vi "obs2lane.vi"(11 "sensors inputs":dbl[][](array[numeric])=[[-2.6493086559458767, 9.313377271515247, 0.316177936945349, -1.2], [-2.6066100840450477, 9.354542103994737, 0.3157590885476819, -1.2], [-2.579340659822815, 9.43207739327695, 0.31450254335468053, -1.2], [-2.6132527619437576, 9.439068677849818, 0.5859163050429868, 1.2000000000000006], [-2.6655003955140795, 9.41719146151926, 0.4953083793337705, 0.40000000000000013], [-2.8189313467074544, 9.344249551531279, 0.5859163050429868, 1.2000000000000006], [-2.5692189092921667, 9.480018973387281, 0.5863351534406539, 1.2000000000000006], [-2.6731933264342116, 9.434269134901442, 0.5863351534406539, 1.2000000000000006], [-2.77635346299322, 9.386711660550553, 0.5863351534406539, 1.2000000000000006], [-2.7290628288714722, 9.419794899689457, 0.5865445776394874, 1.2000000000000006], [-3.035140869949269, 9.26885391372332, 0.5865445776394874, 1.2000000000000006], [-2.550914688564252, 9.509578404068655, 0.3132459981616791, -1.2], [-2.785425991035746, 9.405948172518677, 0.495587629745689, 0.40000000000000013], [-2.7463409502228373, 9.457274042188466, 0.4957970675546278, 0.40000000000000013], [-2.90576588154835, 9.392310316924437, 0.49586688015760744, 0.40000000000000013], [-2.494747129058042, 9.597974241579312, 0.5880105470313224, 1.2000000000000006], [-2.836998990617639, 9.447892074399023, 0.4039934946364334, -0.3999999999999999], [-3.1184925197733824, 9.303796817000539, 0.5880105470313224, 1.2000000000000006], [-2.970577318209098, 9.393517402151646, 0.4960763179665463, 0.40000000000000013], [-2.9699981982750367, 9.392368449256733, 0.588219971230156, 1.2000000000000006], [-3.0729809459427746, 9.340776068194645, 0.4960763179665463, 0.40000000000000013], [-3.1996655181339673, 9.27234939560896, 0.40392368203345375, -0.3999999999999999], [-3.4973819131319495, 9.096981036828707, 0.40392368203345375, -0.3999999999999999], [-2.5289827185611418, 9.605504378157487, 0.3115706045710105, -1.2], [-3.453631348161608, 9.135814142218397, 0.4038538694304742, -0.3999999999999999], [-3.2339632015510937, 9.274656811335685, 0.5886388196278232, 1.2000000000000006], [-2.483097010676977, 9.64588076688389, 0.3111517561733434, -1.2], [-2.8803018639560647, 9.47148380231442, 0.4962857557754851, 0.40000000000000013], [-2.9317308980723027, 9.444962161904348, 0.5888482438266567, 1.2000000000000006], [-2.9582194094409178, 9.433270224287725, 0.4037142442245149, -0.3999999999999999], [-3.0350382771601945, 9.392890956174119, 0.5888482438266567, 1.2000000000000006], [-2.4599617564514022, 9.665942841266034, 0.5890576680254903, 1.2000000000000006], [-3.1930649800894275, 9.320188914278454, 0.5890576680254903, 1.2000000000000006], [-3.424919733239901, 9.200023640728578, 0.4035746190185557, -0.3999999999999999], [-3.4490855593711203, 9.183917089574846, 0.5892670922243238, 1.2000000000000006], [-2.6822275888719656, 9.595825896338217, 0.49649519358442396, 0.40000000000000013], [-3.1777999006997932, 9.352779338748892, 0.40350480641557607, -0.3999999999999999], [-3.3543988506422, 9.251882705008573, 0.5894765164231575, 1.2000000000000006], [-2.4169315260491846, 9.715129108585124, 0.589685940621991, 1.2000000000000006], [-2.4440270491484113, 9.70452412526726, 0.3103140593780091, -1.2], [-2.4445036099706936, 9.705733945395902, 0.40343499381259645, -0.3999999999999999], [-2.8187951120879293, 9.544925625371082, 0.40343499381259645, -0.3999999999999999], [-2.923864294836344, 9.494810195959495, 0.40343499381259645, -0.3999999999999999], [-3.4095769435307015, 9.230983589588824, 0.589685940621991, 1.2000000000000006], [-3.032582634559555, 9.45177853739907, 0.40336518120961684, -0.3999999999999999], [-3.2893092213922506, 9.313834366383366, 0.40336518120961684, -0.3999999999999999], [-3.313999270308597, 9.298296139668594, 0.5898953648208245, 1.2000000000000006], [-2.424651387634039, 9.734980699717582, 0.4967046313933628, 0.40000000000000013], [-2.533097518783729, 9.691715080471495, 0.4967046313933628, 0.40000000000000013], [-2.6407720438905313, 9.646563404831404, 0.4967046313933628, 0.40000000000000013], [-3.4004241638790518, 9.27277469308272, 0.4032255560036576, -0.3999999999999999], [-2.6217419806033297, 9.676437047583807, 0.403155743400678, -0.3999999999999999], [-2.6755410498513874, 9.653323143325384, 0.403155743400678, -0.3999999999999999], [-2.782523848427478, 9.605691332564723, 0.403155743400678, -0.3999999999999999], [-3.072259099823128, 9.465159649093863, 0.496844256599322, 0.40000000000000013], [-3.1500774192579093, 9.424433970288224, 0.403155743400678, -0.3999999999999999], [-3.605192513867668, 9.159018691750026, 0.403155743400678, -0.3999999999999999], [-2.5981277248582337, 9.69583138333276, 0.5907330616161588, 1.2000000000000006], [-3.102875064220138, 9.460567540591395, 0.4030859307976984, -0.3999999999999999], [-3.3599181191701257, 9.319548891673922, 0.4030859307976984, -0.3999999999999999], [-3.385278626883318, 9.304833131837459, 0.49691406920230163, 0.40000000000000013], [-2.5247869108477885, 9.749066890716904, 0.40294630559173916, -0.3999999999999999], [-2.5792234787521573, 9.726796302794572, 0.40294630559173916, -0.3999999999999999], [-3.551164984637863, 9.238618668727831, 0.5913613342126596, 1.2000000000000006], [-2.394482152160173, 9.820127604989409, 0.5915707584114931, 1.2000000000000006], [-2.7494727028492556, 9.675416799445248, 0.40280668038577994, -0.3999999999999999], [-3.681670154810481, 9.169274879714472, 0.40280668038577994, -0.3999999999999999], [-2.349619394154346, 9.868922054648976, 0.5921990310079939, 1.2000000000000006], [-2.625703441413957, 9.761592003343525, 0.497402757423159, 0.40000000000000013], [-3.2137622211581482, 9.48110235361721, 0.497402757423159, 0.40000000000000013], [-3.7275762623275384, 9.185498662423365, 0.5924084552068274, 1.2000000000000006], [-2.3569997188774257, 9.88892730018629, 0.4975423826291182, 0.40000000000000013], [-3.6331178758069624, 9.258143332791025, 0.5926178794056609, 1.2000000000000006], [-3.280263464375405, 9.479130763175284, 0.4976121952320978, 0.40000000000000013], [-2.450699178158054, 9.884289629873633, 0.30675384799783845, -1.2], [-2.4511770399787394, 9.885534502477135, 0.40224817956194303, -0.3999999999999999], [-2.5345511058394776, 9.852902522117958, 0.49775182043805705, 0.40000000000000013], [-3.824786250125524, 9.17047880734031, 0.40224817956194303, -0.3999999999999999], [-2.405397050205525, 9.933526651907876, 0.3061255754013377, -1.2], [-3.4089243051435196, 9.464380504252652, 0.4979612582469959, 0.40000000000000013], [-3.56907303823246, 9.381650335067114, 0.4980310708499755, 0.40000000000000013], [-3.532949127216187, 9.438353586460368, 0.49824050865891434, 0.40000000000000013], [-3.737313762681747, 9.3103050041449, 0.5947121213939967, 1.2000000000000006], [-2.2908474536598415, 10.059979664182297, 0.595549818189331, 1.2000000000000006], [-2.3765186719612967, 10.02943138812595, 0.3044501818106692, -1.2], [-2.462262709016492, 9.999031326649108, 0.4985197590708328, 0.40000000000000013], [-3.657097646318684, 9.409803942456133, 0.4985197590708328, 0.40000000000000013], [-3.835868568229564, 9.295365230962426, 0.40148024092916723, -0.3999999999999999], [-2.3581413988349413, 10.067967806625958, 0.5961780907858316, 1.2000000000000006], [-3.877029743260587, 9.302385055789298, 0.5961780907858316, 1.2000000000000006], [-3.9331436519651666, 9.276595165706414, 0.5963875149846652, 1.2000000000000006], [-3.425151432335213, 9.616047962173518, 0.4989386346887105, 0.40000000000000013], [-2.3143719287589564, 10.127343415537375, 0.49900844729169014, 0.40000000000000013], [-3.7975482431761254, 9.403949992407117, 0.49900844729169014, 0.40000000000000013], [-3.854407472044735, 9.378948406292697, 0.49907825989466975, 0.40000000000000013], [-2.407763132093687, 10.115274836822742, 0.4008519275023507, -0.3999999999999999], [-2.468901871015975, 10.10337801061548, 0.4007821148993711, -0.3999999999999999], [-2.3890129763037065, 10.15395227178771, 0.4993575103065882, 0.40000000000000013], [-3.777898705712374, 9.487607060347795, 0.4994273229095678, 0.40000000000000013], [-4.0346920104398265, 9.315984499311078, 0.5982723327741674, 1.2000000000000006], [-4.015722357091047, 9.342912286209264, 0.40050286448745265, -0.3999999999999999], [-2.372846250599384, 10.200711102617147, 0.30109939462933205, -1.2], [-2.3833228936159903, 10.23029622982958, 0.4001538014725545, -0.3999999999999999], [-3.9666747963375277, 9.4365483588187, 0.4998461985274455, 0.40000000000000013], [-2.30100181314674, 10.278532756817912, 0.5999477263648358, 1.2000000000000006], [-4.109576508398126, 9.423930057048132, 0.5003348867483028, 0.40000000000000013], [-2.35334151682133, 10.334600032038626, 0.2985863042433292, -1.2], [-4.074608378760497, 9.48436394539886, 0.5005443245572416, 0.40000000000000013], [-2.3368079650044735, 10.384014278769136, 0.5007537623661805, 0.40000000000000013], [-2.370078405901655, 10.38320748736416, 0.39917642503083994, -0.3999999999999999], [-4.204212822255533, 9.504238162023881, 0.3988273620159418, -0.3999999999999999], [-2.2707767805352264, 10.48873231405309, 0.2960732138573263, -1.2], [-2.3200348724405737, 10.53572713543776, 0.6051833313356751, 1.2000000000000006], [-2.245779677656643, 10.622703152908741, 0.29356012347132354, -1.2], [-2.279884830624796, 10.622358187824348, 0.6066493007275101, 1.2000000000000006], [-2.358065997017253, 10.651060149761754, 0.5025688900436505, 0.40000000000000013], [-2.206922249961846, 10.718517420078616, 0.29188472988065495, -1.2], [-2.310815072326706, 10.718984235455277, 0.5029179530585486, 0.40000000000000013], [-2.250256927274077, 10.7470116403635, 0.6089529669146794, 1.2000000000000006], [-2.4078141528407944, 10.696197951674801, 0.2910470330853207, -1.2], [-2.2625570787999116, 10.786624601979373, 0.5032670160734467, 0.40000000000000013], [-2.37319268235858, 10.803936049039782, 0.3963839209116553, -0.3999999999999999], [-2.4400133449020482, 10.792431192800741, 0.3963141083086757, -0.3999999999999999], [-2.3484550625403937, 10.948347869936686, 0.3954763570729203, -0.3999999999999999], [-2.2532005442925973, 10.986565753726355, 0.6137697234878515, 1.2000000000000006], [-2.2241527610867795, 11.130722431723722, 0.6164922380726879, 1.2000000000000006], [-2.3272220554510197, 11.112000353866012, 0.3944291680282261, -0.3999999999999999], [-2.2968682826047866, 11.131657762965752, 0.5056406445747536, 0.40000000000000013], [-2.2805508875817773, 11.32421563798276, 0.5068972714283867, 0.40000000000000013], [-2.3203488195890745, 11.3333663356091, 0.39296310336565415, -0.3999999999999999], [-2.2253235316083524, 11.390402063747686, 0.6217278430435271, 1.2000000000000006], [-2.23390046248441, 11.420813566670208, 0.5074557722522236, 0.40000000000000013], [-2.315297365324197, 11.574401473618405, 0.391357413497123, -0.3999999999999999], [-2.2168668356954866, 11.63137340411444, 0.6265445996166993, 1.2000000000000006], [-2.3994033185138965, 11.600249851280598, 0.2730365519856337, -1.2], [-2.233080590823236, 11.690844769333019, 0.5092708999296937, 0.40000000000000013], [-2.3589382981537037, 11.726595493110718, 0.27073288579846444, -1.2], [-2.3008663461775223, 11.796656013544418, 0.38989134883455107, -0.3999999999999999], [-2.209460232985442, 11.892117815907735, 0.6317802045875385, 1.2000000000000006], [-2.2516708194251622, 11.903349900014954, 0.3892630354077345, -0.3999999999999999], [-2.324463966690179, 11.881746284197003, 0.26780094701479445, -1.2], [-2.2175289279374653, 11.922764866099948, 0.5108067771952451, 0.40000000000000013], [-2.2538194745555633, 11.911368790129554, 0.2675915228159609, -1.2], [-2.178403555854863, 12.077484518563601, 0.5117841536369597, 0.40000000000000013], [-2.1829008579162608, 12.095192687788384, 0.6357592643653763, 1.2000000000000006], [-2.2383426880850124, 12.155028982889158, 0.3875875329362237, -0.3999999999999999], [-2.2804615843118747, 12.317890670472249, 0.25921455486261813, -1.2], [-2.2227746224162255, 12.415062075134333, 0.2575391612719496, -1.2], [-2.186230627716147, 12.434387153701119, 0.6426702629268841, 1.2000000000000006], [-2.196164124819029, 12.474982005763925, 0.5145068451531648, 0.40000000000000013], [-2.1425536546232067, 12.599100045840768, 0.6458116259093877, 1.2000000000000006], [-2.2643337612516414, 12.581746676789589, 0.3846554036110799, -0.3999999999999999], [-2.198573038349574, 12.65771577116447, 0.2527224046987775, -1.2], [-2.1750587039156537, 12.73714405461915, 0.5162521602276552, 0.40000000000000013], [-2.238686482838199, 12.824800292270476, 0.38304971374254876, -0.3999999999999999], [-2.1747996213790666, 12.920092091405744, 0.24748679972793824, -1.2], [-2.1535345564869504, 13.01725329936264, 0.6543980180615641, 1.2000000000000006], [-2.187058282696622, 13.165406851352257, 0.519184289552799, 0.40000000000000013], [-2.0682676188644926, 13.230434114169201, 0.24162292216059827, -1.2], [-2.249455724453499, 13.24346320074072, 0.3801873970203845, -0.3999999999999999], [-2.168249294443763, 13.280340530506738, 0.2401569527687633, -1.2], [-2.1361605605328022, 13.338559010168616, 0.6608901682254047, 1.2000000000000006], [-2.1577943406236098, 13.438198159944571, 0.520999417230269, 0.40000000000000013], [-2.1011219599138715, 13.601533356858653, 0.6661257731962439, 1.2000000000000006], [-2.2400954133839512, 13.604417430165359, 0.377743955916098, -0.3999999999999999], [-2.1622288912277443, 13.672487145254262, 0.3773948929011999, -0.3999999999999999], [-2.0809447496291567, 13.728170217410458, 0.23136113641775338, -1.2], [-2.148368119037393, 13.828678025980699, 0.5236522961434944, 0.40000000000000013], [-2.1431530665836362, 14.033933863880375, 0.37495145179691336, -0.3999999999999999], [-2.106513383233814, 14.090157922222986, 0.6761781347402553, 1.2000000000000006], [-2.116678410658171, 14.141260966031997, 0.5257466742328829, 0.40000000000000013], [-2.0736923856429295, 14.42245242291376, 0.6828797091029295, 1.2000000000000006], [-2.0946138788714483, 14.532649102029193, 0.5283995531461083, 0.40000000000000013], [-2.152273017194013, 14.572484794069997, 0.3712513838389937, -0.3999999999999999], [-2.0231688076393577, 14.688270075344283, 0.5293769295878229, 0.40000000000000013], [-2.0756120529212976, 14.699000478760663, 0.37048344520621795, -0.3999999999999999], [-2.0476810196035475, 14.823824383301131, 0.6910472528574387, 1.2000000000000006], [8.784462172926562, 11.47924364037722, 0.6985865240154472, 1.2000000000000006], [8.643867253715156, 11.631338367097312, 0.6985865240154472, 1.2000000000000006], [-2.01182307782236, 15.20812065601524, 0.5329373723397832, 0.40000000000000013], [8.86867671544905, 11.41559660678595, 0.6990053724131143, 1.2000000000000006], [8.58702381954077, 11.72028699299172, 0.6990053724131143, 1.2000000000000006], [8.952448256526495, 11.35108640713428, 0.6994242208107815, 1.2000000000000006], [8.751204607664915, 11.589530329880938, 0.699633645009615, 1.2000000000000006], [-2.0698358361213067, 15.238622346987988, 0.36678337724829835, -0.3999999999999999], [8.78228318958885, 11.618259075505645, 0.5334958731636202, 0.40000000000000013], [9.066064089233228, 11.311820599800757, 0.7006807660037829, 1.2000000000000006], [8.586576710391817, 11.864672700124274, 0.7010996144014501, 1.2000000000000006], [8.904607069385332, 11.588375580628155, 0.5339845613844775, 0.40000000000000013], [8.9823118978036, 11.517019884769494, 0.5340543739874571, 0.40000000000000013], [-2.038520846959818, 15.363492520347437, 0.7021467353956179, 1.2000000000000006], [8.791223365347536, 11.769957155305526, 0.5342638117963959, 0.40000000000000013], [8.577157812432615, 12.002632694506751, 0.7029844321909522, 1.2000000000000006], [9.089521761789143, 11.471296644949536, 0.5344034370023552, 0.40000000000000013], [8.747614402156172, 11.874019031613333, 0.5345430622083145, 0.40000000000000013], [9.196614789945517, 11.42431028033962, 0.5347525000172533, 0.40000000000000013], [8.702856524966558, 11.977947480441758, 0.5348223126202329, 0.40000000000000013], [8.551902917074258, 12.126859885849031, 0.7044504015827872, 1.2000000000000006], [9.301763328727434, 11.37452391977877, 0.7052880983781215, 1.2000000000000006], [8.546058430068586, 12.272774370500398, 0.7065446435711229, 1.2000000000000006], [8.713762205484503, 12.13805016075561, 0.5356600638559883, 0.40000000000000013], [9.379898466547676, 11.440670196564861, 0.5357996890619475, 0.40000000000000013], [8.680290014842434, 12.256372289618902, 0.536078939473866, 0.40000000000000013], [-1.9947666269032363, 15.748326418663561, 0.5366374402977029, 0.40000000000000013], [5.4033137061696035, 14.702228724352713, 0.7105237033489606, 1.2000000000000006], [5.31065139179097, 14.760192151279867, 0.5369166907096213, 0.40000000000000013], [5.318145573506214, 14.776082090179019, 0.7111519759454614, 1.2000000000000006], [5.372647557345696, 14.763989846509837, 0.36287387148143985, -0.3999999999999999], [5.430433378499369, 14.758453624273042, 0.5372657537245195, 0.40000000000000013], [5.282599535397169, 14.828571261939807, 0.3627342462754806, -0.3999999999999999], [-2.0630447970868317, 15.828269580660534, 0.3627342462754806, -0.3999999999999999], [-2.0425899368277762, 16.04197255374355, 0.7161781567174671, 1.2000000000000006], [8.986023479525567, 16.697743175440838, 0.7844504455372108, 1.2000000000000006], [8.870510744967275, 16.775657498704163, 0.7844504455372108, 1.2000000000000006], [8.776249405862337, 16.886004939029128, 0.7852881423325451, 1.2000000000000006], [9.255378545456706, 16.596057732863006, 0.7859164149290457, 1.2000000000000006], [9.146441633836046, 16.684541131912827, 0.7861258391278794, 1.2000000000000006], [9.094705994581439, 16.85736482840408, 0.5628171664150587, 0.40000000000000013], [9.445245140600367, 16.620273164434607, 0.7886389295138823, 1.2000000000000006], [8.745638718171325, 17.096618222434593, 0.7886389295138823, 1.2000000000000006], [9.250822015437112, 16.835004830220694, 0.563305854635916, 0.40000000000000013], [8.898582257650931, 17.072593546817984, 0.563305854635916, 0.40000000000000013], [9.372609476756939, 16.761935663932476, 0.5633756672388956, 0.40000000000000013], [9.022240713238299, 17.00273744358763, 0.5633756672388956, 0.40000000000000013], [9.671704217358442, 16.690540187776413, 0.79261798929172, 1.2000000000000006], [8.733353836557999, 17.341528099528503, 0.7928274134905535, 1.2000000000000006], [9.575618663038583, 16.801373411419853, 0.5644228562835899, 0.40000000000000013], [8.86635551362631, 17.284293500790973, 0.5644228562835899, 0.40000000000000013], [-11.730647795102412, 15.437193920648374, 0.09942389115260453, -1.2], [-11.753961919567294, 15.46091854606451, 0.3329242648031848, -0.3999999999999999], [-2.6376199176507695, 22.880864643377365, 0.586553451428128, 0.40000000000000013], [-2.8095170709695823, 22.87690194098971, 0.5866930766340872, 0.40000000000000013], [-2.472177558679492, 22.932903386537202, 0.5867628892370669, 0.40000000000000013], [-2.1457138125258957, 23.092372962417727, 0.5876006404728222, 0.40000000000000013], [-1.975660428365826, 23.120301035359756, 0.5876704530758019, 0.40000000000000013], [-2.830488522803034, 23.021539526550544, 0.8631939442986329, 1.2000000000000006], [-2.321307029798844, 23.112624067398425, 0.5878798908847407, 0.40000000000000013], [-2.664069979468923, 23.075216022238337, 0.8638222168951337, 1.2000000000000006], [-2.4981915740055283, 23.137390254704062, 0.864659913690468, 1.2000000000000006], [-2.3314305321547493, 23.198157106933053, 0.8654976104858023, 1.2000000000000006], [-1.8217528316749911, 23.325992950774253, 0.5889968925324145, 0.40000000000000013], [-2.1768599709453524, 23.37676650480826, 0.8688483976671393, 1.2000000000000006], [-15.001217509405912, 16.7719561296704, 0.31016535623183017, -0.3999999999999999], [-15.131558329077535, 16.65366297795977, 0.31002573102587094, -0.3999999999999999], [-14.921984448489132, 16.935815146369087, 0.30981629321693205, -0.3999999999999999], [-15.241790010790758, 16.749485916960253, 0.026963118356189475, -1.2], [-15.133075455565274, 16.88861418597005, 0.0267536941573559, -1.2], [-15.017973364486107, 17.261437164441947, 0.3077917277305232, -0.3999999999999999], [9.64601974480163, 21.452115753566822, 0.5922780848724565, 0.40000000000000013], [9.496453028675626, 21.54978831901161, 0.8772253656204823, 1.2000000000000006], [9.33857931433906, 21.631972172843444, 0.8772253656204823, 1.2000000000000006], [9.17999443103193, 21.712775206793534, 0.8772253656204823, 1.2000000000000006], [-15.156829567346312, 17.1472706411717, 0.022774634379518044, -1.2], [9.377029264437805, 21.70662736414938, 0.5929762109022526, 0.40000000000000013], [9.544865059367709, 21.641804454240944, 0.5931158361082118, 0.40000000000000013], [9.710389454590258, 21.571913609233842, 0.8797384560064849, 1.2000000000000006], [-1.8772014233671248, 23.929435618135358, 0.8797384560064849, 1.2000000000000006], [9.095883042737146, 21.944626194626313, 0.8807855770006529, 1.2000000000000006], [9.271801932592034, 21.894917952170292, 0.5938139621380081, 0.40000000000000013], [-15.236180272734178, 17.461386956855613, 0.017120181011011648, -1.2], [9.194957789557106, 22.145529906980062, 0.5951404015946207, 0.40000000000000013], [5.3379716006680615, 24.14040468850077, 0.30115953044745974, -0.3999999999999999], [5.346343602955266, 24.94301298686431, 0.29571414741504976, -0.3999999999999999], [-16.03827076279453, 20.400810973707614, 0.28733663505749585, -0.3999999999999999], [-15.917453817284267, 20.56937941691859, 0.2870573846455774, -0.3999999999999999], [-15.794914133758107, 20.737124067829413, 0.28677813423365894, -0.3999999999999999], [-14.857892347507073, 21.847969012040384, 0.2851724443651278, -0.3999999999999999], [-15.023801434595246, 21.725328510394597, 0.2851026317621482, -0.3999999999999999], [-15.339589077483758, 21.460351215716504, 0.2851026317621482, -0.3999999999999999], [-15.650704132941332, 21.189903024072276, 0.2851026317621482, -0.3999999999999999], [-15.201556508849778, 21.61650958244562, 0.28489319395320933, -0.3999999999999999], [-14.728337374906722, 22.016057756865447, 0.2848233813502297, -0.3999999999999999], [-15.626945243640977, 21.4767441096572, 0.28370637970255586, -0.3999999999999999], [9.50763508171292, 26.73975570562619, 0.6252994460818146, 0.40000000000000013], [-1.4252219468434035, 28.59895493907886, 0.6255088838907534, 0.40000000000000013], [9.725543674751258, 26.692789231824694, 0.6255786964937331, 0.40000000000000013], [9.943355423856874, 26.64378657215293, 0.6258579469056516, 0.40000000000000013], [9.334114379546264, 26.89614247546073, 0.6258579469056516, 0.40000000000000013], [9.216574706656742, 27.200382540182076, 0.6275334493771623, 0.40000000000000013], [10.040081267648652, 26.868922071117122, 0.9827751618326013, 1.2000000000000006], [-1.4946609322957394, 29.821814277404098, 1.0022516123241232, 1.2000000000000006], [9.883884675811041, 31.803099088007194, 0.6592981837328874, 0.40000000000000013], [9.665449175747526, 31.97349509801759, 0.659926497159704, 0.40000000000000013], [10.174424429491456, 31.838119222564067, 0.6602057475716224, 0.40000000000000013], [10.17244090528941, 31.83259465007272, 1.0805762626878783, 1.2000000000000006], [-1.0364518801246452, 37.42334336490329, 0.6869439745128152, 0.40000000000000013], [10.026103833352638, 36.8130958059697, 0.6928780457660825, 0.40000000000000013], [9.743408822772697, 36.92812129013003, 0.6930874835750214, 0.40000000000000013], [10.347031193921643, 36.82288619877287, 1.1808904539291583, 1.2000000000000006], [-21.069030510629236, 31.45954783569295, 0.20558607696836614, -0.3999999999999999], [-21.391355310423045, 31.377757000004777, 0.20467851312963112, -0.3999999999999999], [10.4210427571751, 41.72394225688742, 0.7265975330052368, 0.40000000000000013], [10.107451026305094, 41.89078819565647, 0.7271560338290737, 0.40000000000000013], [10.474235594988285, 41.919051326913184, 1.284136583954108, 1.2000000000000006], [10.13857155297352, 42.00899223589921, 1.284136583954108, 1.2000000000000006], [10.830210018606069, 41.90102810572798, 0.7285522858886659, 0.40000000000000013], [-0.709038750028526, 57.66347671663537, 1.5846603092802805, 1.2000000000000006], [11.120605021860856, 56.96437033164037, 0.8312466248716806, 0.40000000000000013], [-0.7151980727209852, 58.133987434462625, 0.8314560626806193, 0.40000000000000013], [1.5195348183779678, 61.52869356204023, 0.04473783970333195, -0.3999999999999999], [5.073212151726797, 61.48708023724171, 0.04362083805565814, -0.3999999999999999], [11.439817695944253, 61.011847285540675, 0.8593811038724656, 0.40000000000000013], [11.689176472740309, 65.06866600393317, 0.8875155828732506, 0.40000000000000013], [14.49832831315618, 65.07219891982305, 1.7750269060199955, 1.2000000000000006], [8.818111571073048, 72.81602044955893, 1.9136657256478184, 1.2000000000000006], [12.551831810983316, 72.91253923612891, 0.9424581014182081, 0.40000000000000013], [13.768405529858791, 72.71844886386302, 1.9283254195661683, 1.2000000000000006], [1.2476421313017925, 74.97736983119862, -0.04909029870127124, -0.3999999999999999], [0.9387629168292289, 75.21210795753403, 0.9506959885698028, 0.40000000000000013], [17.77975821366545, 76.1598746565128, 2.0169118556727685, 1.2000000000000006], [47.35648972259149, 63.571420836353425, 2.052304545275642, 1.2000000000000006], [13.031972557350265, 79.3416128979354, 2.061938058421986, 1.2000000000000006], [24.83184721270082, 81.07466865802802, 2.156178947897092, 1.2000000000000006], [13.551875448365177, 86.71163580640813, 1.0385900557211387, 0.40000000000000013], [52.872675769586, 69.37798867554798, 2.2194250559448303, 1.2000000000000006], [8.915518332671137, 92.0400907270114, 1.0712623539155988, 0.40000000000000013], [9.692181670683942, 91.99867908899289, 1.0715416043275172, 0.40000000000000013], [20.71894414488982, 95.06455786989261, 2.4164932270472192, 1.2000000000000006], [19.150342204408794, 95.56882049865551, 2.4198440142285564, 1.2000000000000006], [23.490178905085354, 95.9928006820069, 2.448953977866423, 1.2000000000000006], [26.036285319817722, 95.81770414584793, 2.4592157636092677, 1.2000000000000006], [14.717578948116746, 99.12164584891, 1.1254369338277803, 0.40000000000000013], [20.65463162219833, 155.2673630873944, 3.658378726130288, 1.2000000000000006], [12.312708261276875, 191.3556263648354, 4.393457664036117, 1.2000000000000006], [14.978259637770336, 232.0240814937235, 2.048848233439155, 0.40000000000000013], [33.73593705129936, 288.53349296533526, 2.4538311433239053, 0.40000000000000013], [8.92096999050232, 17.23708913161584, 0.3356469563193898, -0.3999999999999999], [-2.5256202703736608, 22.68399055587274, 0.31491261323444397, -0.3999999999999999], [-1.8996165215080512, 23.228271875851924, 0.3116314208944021, -0.3999999999999999], [-3.0296332585078587, 23.183843349397314, 0.8671730040764709, 1.2000000000000006], [5.104128617356655, 23.236200962780366, 0.022984058578351618, -1.2], [-1.2548826959515347, 24.01715071826592, 0.01942384719818102, -1.2], [5.221948215230284, 24.444090337557157, -0.0021468452816766903, -1.2], [-2.224688830349968, 25.593404278777417, 0.9151311456093583, 1.2000000000000006], [5.209357772395169, 25.198536731676327, -0.017434811796527283, -1.2], [-1.1725915542855405, 25.874379726198075, -0.019319629586029397, -1.2], [-15.005798944565672, 21.383214801932546, -0.039005504276384995, -1.2], [-14.976356804490646, 21.66777357175441, -0.04319398825305637, -1.2], [-14.955664951264778, 21.9687081224078, -0.04780132062739484, -1.2], [9.275033221452706, 26.45651279141699, 0.277143995022472, -0.3999999999999999], [9.363878146139614, 27.271589550954324, 0.2716287993870824, -0.3999999999999999], [9.371321144452127, 28.564736959442584, 0.26318147442654893, -0.3999999999999999], [10.747513637749273, 30.43885569655537, 1.0575396008161857, 1.2000000000000006], [11.012472531760006, 30.418068389611857, 1.0592149944068543, 1.2000000000000006], [11.266285997376329, 30.367042635463775, 1.060262115401022, 1.2000000000000006], [-20.735017036098906, 31.521767273772653, 0.20663326601306034, -0.3999999999999999], [-20.49557227262787, 31.709735125755284, 0.20656345341008076, -0.3999999999999999], [10.724864676049275, 37.00446773130826, 0.6956007372822874, 0.40000000000000013], [-21.806198041420327, 31.41066071306105, 0.20272376024620187, -0.3999999999999999], [10.97816933233072, 46.72664514439962, 0.7613642092890853, 0.40000000000000013], [-33.95444016665767, 37.454440166657676, 0.11475988049188635, -0.3999999999999999], [-33.46782468155926, 38.15694699438283, 0.11364287884421248, -0.3999999999999999], [-32.258000408687934, 39.32613895725404, 0.11343344103527364, -0.3999999999999999], [-34.39923085728631, 37.30403001674005, 0.11329381582931441, -0.3999999999999999], [11.618566184124763, 57.01187131155995, 0.8322938139163747, 0.40000000000000013], [16.615400312068406, 60.50485600252477, 1.6937703168725702, 1.2000000000000006], [13.205163345895427, 64.3192947748755, 1.7536656377389712, 1.2000000000000006], [20.538690765112868, 64.00503191176435, 1.7884300547453438, 1.2000000000000006], [13.026046392769018, 79.30712465157343, 0.9869985421192027, 0.40000000000000013], [27.29899080749756, 81.67230442986731, 2.1844512147396244, 1.2000000000000006], [33.69042505267091, 80.06731529671714, 2.2022522716404778, 1.2000000000000006], [29.157427120978678, 82.5346645544511, 2.2146082993716583, 1.2000000000000006], [27.17382907061827, 93.78874887901951, 2.425079619199396, 1.2000000000000006], [34.761055666251615, 92.88790635480824, 2.4590063394104344, 1.2000000000000006], [-2.729118001525531, 22.918683596868465, 0.31309748555697403, -0.3999999999999999], [9.124522914489708, 21.80096170236561, 0.3072332269066863, -0.3999999999999999], [-1.5170192378515415, 28.303045293335575, 0.2765156815956554, -0.3999999999999999], [-1.3900091234452605, 30.022954081648294, 0.2645777264861412, -0.3999999999999999], [4.034616118215339, 61.19769858054814, 0.04620390436590388, -0.3999999999999999], [26.121526235859253, 82.71602090547535, 2.197226090868472, 1.2000000000000006]]) -> ()   [LabVIEW 2012]
uses:
  G_SEN.vi
  <vilib>/Analysis/Matrix/Numeric/Conversions/Array To Matrix - RA2.vi
  <vilib>/Analysis/baseanly.llb/Real Inverse Matrix.vi
  <vilib>/Analysis/baseanly.llb/A x Vector.vi
  <vilib>/Analysis/Matrix/NI_Matrix.lvlib
  <vilib>/Analysis/NI_AALBase.lvlib
panel:
  in  "Numeric":dbl=0.8
  in  "lane num":i32=6
  in  "order":i32=2 min=0 max=2 step=1
  out "Array":dbl[](array[numeric])
  out "Array 2":i16[](array[numeric])
  out "time":u32
  out "lanes":dbl[][](array[numeric])
  out "lane_x":dbl[](array[numeric])
  out "sensors":dbl[][](array[numeric])=[[-2.6493086559458767, 9.313377271515247, 0.316177936945349, -1.2], [-2.6066100840450477, 9.354542103994737, 0.3157590885476819, -1.2], [-2.579340659822815, 9.43207739327695, 0.31450254335468053, -1.2], [-2.6132527619437576, 9.439068677849818, 0.5859163050429868, 1.2000000000000006], [-2.6655003955140795, 9.41719146151926, 0.4953083793337705, 0.40000000000000013], [-2.8189313467074544, 9.344249551531279, 0.5859163050429868, 1.2000000000000006], [-2.5692189092921667, 9.480018973387281, 0.5863351534406539, 1.2000000000000006], [-2.6731933264342116, 9.434269134901442, 0.5863351534406539, 1.2000000000000006], [-2.77635346299322, 9.386711660550553, 0.5863351534406539, 1.2000000000000006], [-2.7290628288714722, 9.419794899689457, 0.5865445776394874, 1.2000000000000006], [-3.035140869949269, 9.26885391372332, 0.5865445776394874, 1.2000000000000006], [-2.550914688564252, 9.509578404068655, 0.3132459981616791, -1.2], [-2.785425991035746, 9.405948172518677, 0.495587629745689, 0.40000000000000013], [-2.7463409502228373, 9.457274042188466, 0.4957970675546278, 0.40000000000000013], [-2.90576588154835, 9.392310316924437, 0.49586688015760744, 0.40000000000000013], [-2.494747129058042, 9.597974241579312, 0.5880105470313224, 1.2000000000000006], [-2.836998990617639, 9.447892074399023, 0.4039934946364334, -0.3999999999999999], [-3.1184925197733824, 9.303796817000539, 0.5880105470313224, 1.2000000000000006], [-2.970577318209098, 9.393517402151646, 0.4960763179665463, 0.40000000000000013], [-2.9699981982750367, 9.392368449256733, 0.588219971230156, 1.2000000000000006], [-3.0729809459427746, 9.340776068194645, 0.4960763179665463, 0.40000000000000013], [-3.1996655181339673, 9.27234939560896, 0.40392368203345375, -0.3999999999999999], [-3.4973819131319495, 9.096981036828707, 0.40392368203345375, -0.3999999999999999], [-2.5289827185611418, 9.605504378157487, 0.3115706045710105, -1.2], [-3.453631348161608, 9.135814142218397, 0.4038538694304742, -0.3999999999999999], [-3.2339632015510937, 9.274656811335685, 0.5886388196278232, 1.2000000000000006], [-2.483097010676977, 9.64588076688389, 0.3111517561733434, -1.2], [-2.8803018639560647, 9.47148380231442, 0.4962857557754851, 0.40000000000000013], [-2.9317308980723027, 9.444962161904348, 0.5888482438266567, 1.2000000000000006], [-2.9582194094409178, 9.433270224287725, 0.4037142442245149, -0.3999999999999999], [-3.0350382771601945, 9.392890956174119, 0.5888482438266567, 1.2000000000000006], [-2.4599617564514022, 9.665942841266034, 0.5890576680254903, 1.2000000000000006], [-3.1930649800894275, 9.320188914278454, 0.5890576680254903, 1.2000000000000006], [-3.424919733239901, 9.200023640728578, 0.4035746190185557, -0.3999999999999999], [-3.4490855593711203, 9.183917089574846, 0.5892670922243238, 1.2000000000000006], [-2.6822275888719656, 9.595825896338217, 0.49649519358442396, 0.40000000000000013], [-3.1777999006997932, 9.352779338748892, 0.40350480641557607, -0.3999999999999999], [-3.3543988506422, 9.251882705008573, 0.5894765164231575, 1.2000000000000006], [-2.4169315260491846, 9.715129108585124, 0.589685940621991, 1.2000000000000006], [-2.4440270491484113, 9.70452412526726, 0.3103140593780091, -1.2], [-2.4445036099706936, 9.705733945395902, 0.40343499381259645, -0.3999999999999999], [-2.8187951120879293, 9.544925625371082, 0.40343499381259645, -0.3999999999999999], [-2.923864294836344, 9.494810195959495, 0.40343499381259645, -0.3999999999999999], [-3.4095769435307015, 9.230983589588824, 0.589685940621991, 1.2000000000000006], [-3.032582634559555, 9.45177853739907, 0.40336518120961684, -0.3999999999999999], [-3.2893092213922506, 9.313834366383366, 0.40336518120961684, -0.3999999999999999], [-3.313999270308597, 9.298296139668594, 0.5898953648208245, 1.2000000000000006], [-2.424651387634039, 9.734980699717582, 0.4967046313933628, 0.40000000000000013], [-2.533097518783729, 9.691715080471495, 0.4967046313933628, 0.40000000000000013], [-2.6407720438905313, 9.646563404831404, 0.4967046313933628, 0.40000000000000013], [-3.4004241638790518, 9.27277469308272, 0.4032255560036576, -0.3999999999999999], [-2.6217419806033297, 9.676437047583807, 0.403155743400678, -0.3999999999999999], [-2.6755410498513874, 9.653323143325384, 0.403155743400678, -0.3999999999999999], [-2.782523848427478, 9.605691332564723, 0.403155743400678, -0.3999999999999999], [-3.072259099823128, 9.465159649093863, 0.496844256599322, 0.40000000000000013], [-3.1500774192579093, 9.424433970288224, 0.403155743400678, -0.3999999999999999], [-3.605192513867668, 9.159018691750026, 0.403155743400678, -0.3999999999999999], [-2.5981277248582337, 9.69583138333276, 0.5907330616161588, 1.2000000000000006], [-3.102875064220138, 9.460567540591395, 0.4030859307976984, -0.3999999999999999], [-3.3599181191701257, 9.319548891673922, 0.4030859307976984, -0.3999999999999999], [-3.385278626883318, 9.304833131837459, 0.49691406920230163, 0.40000000000000013], [-2.5247869108477885, 9.749066890716904, 0.40294630559173916, -0.3999999999999999], [-2.5792234787521573, 9.726796302794572, 0.40294630559173916, -0.3999999999999999], [-3.551164984637863, 9.238618668727831, 0.5913613342126596, 1.2000000000000006], [-2.394482152160173, 9.820127604989409, 0.5915707584114931, 1.2000000000000006], [-2.7494727028492556, 9.675416799445248, 0.40280668038577994, -0.3999999999999999], [-3.681670154810481, 9.169274879714472, 0.40280668038577994, -0.3999999999999999], [-2.349619394154346, 9.868922054648976, 0.5921990310079939, 1.2000000000000006], [-2.625703441413957, 9.761592003343525, 0.497402757423159, 0.40000000000000013], [-3.2137622211581482, 9.48110235361721, 0.497402757423159, 0.40000000000000013], [-3.7275762623275384, 9.185498662423365, 0.5924084552068274, 1.2000000000000006], [-2.3569997188774257, 9.88892730018629, 0.4975423826291182, 0.40000000000000013], [-3.6331178758069624, 9.258143332791025, 0.5926178794056609, 1.2000000000000006], [-3.280263464375405, 9.479130763175284, 0.4976121952320978, 0.40000000000000013], [-2.450699178158054, 9.884289629873633, 0.30675384799783845, -1.2], [-2.4511770399787394, 9.885534502477135, 0.40224817956194303, -0.3999999999999999], [-2.5345511058394776, 9.852902522117958, 0.49775182043805705, 0.40000000000000013], [-3.824786250125524, 9.17047880734031, 0.40224817956194303, -0.3999999999999999], [-2.405397050205525, 9.933526651907876, 0.3061255754013377, -1.2], [-3.4089243051435196, 9.464380504252652, 0.4979612582469959, 0.40000000000000013], [-3.56907303823246, 9.381650335067114, 0.4980310708499755, 0.40000000000000013], [-3.532949127216187, 9.438353586460368, 0.49824050865891434, 0.40000000000000013], [-3.737313762681747, 9.3103050041449, 0.5947121213939967, 1.2000000000000006], [-2.2908474536598415, 10.059979664182297, 0.595549818189331, 1.2000000000000006], [-2.3765186719612967, 10.02943138812595, 0.3044501818106692, -1.2], [-2.462262709016492, 9.999031326649108, 0.4985197590708328, 0.40000000000000013], [-3.657097646318684, 9.409803942456133, 0.4985197590708328, 0.40000000000000013], [-3.835868568229564, 9.295365230962426, 0.40148024092916723, -0.3999999999999999], [-2.3581413988349413, 10.067967806625958, 0.5961780907858316, 1.2000000000000006], [-3.877029743260587, 9.302385055789298, 0.5961780907858316, 1.2000000000000006], [-3.9331436519651666, 9.276595165706414, 0.5963875149846652, 1.2000000000000006], [-3.425151432335213, 9.616047962173518, 0.4989386346887105, 0.40000000000000013], [-2.3143719287589564, 10.127343415537375, 0.49900844729169014, 0.40000000000000013], [-3.7975482431761254, 9.403949992407117, 0.49900844729169014, 0.40000000000000013], [-3.854407472044735, 9.378948406292697, 0.49907825989466975, 0.40000000000000013], [-2.407763132093687, 10.115274836822742, 0.4008519275023507, -0.3999999999999999], [-2.468901871015975, 10.10337801061548, 0.4007821148993711, -0.3999999999999999], [-2.3890129763037065, 10.15395227178771, 0.4993575103065882, 0.40000000000000013], [-3.777898705712374, 9.487607060347795, 0.4994273229095678, 0.40000000000000013], [-4.0346920104398265, 9.315984499311078, 0.5982723327741674, 1.2000000000000006], [-4.015722357091047, 9.342912286209264, 0.40050286448745265, -0.3999999999999999], [-2.372846250599384, 10.200711102617147, 0.30109939462933205, -1.2], [-2.3833228936159903, 10.23029622982958, 0.4001538014725545, -0.3999999999999999], [-3.9666747963375277, 9.4365483588187, 0.4998461985274455, 0.40000000000000013], [-2.30100181314674, 10.278532756817912, 0.5999477263648358, 1.2000000000000006], [-4.109576508398126, 9.423930057048132, 0.5003348867483028, 0.40000000000000013], [-2.35334151682133, 10.334600032038626, 0.2985863042433292, -1.2], [-4.074608378760497, 9.48436394539886, 0.5005443245572416, 0.40000000000000013], [-2.3368079650044735, 10.384014278769136, 0.5007537623661805, 0.40000000000000013], [-2.370078405901655, 10.38320748736416, 0.39917642503083994, -0.3999999999999999], [-4.204212822255533, 9.504238162023881, 0.3988273620159418, -0.3999999999999999], [-2.2707767805352264, 10.48873231405309, 0.2960732138573263, -1.2], [-2.3200348724405737, 10.53572713543776, 0.6051833313356751, 1.2000000000000006], [-2.245779677656643, 10.622703152908741, 0.29356012347132354, -1.2], [-2.279884830624796, 10.622358187824348, 0.6066493007275101, 1.2000000000000006], [-2.358065997017253, 10.651060149761754, 0.5025688900436505, 0.40000000000000013], [-2.206922249961846, 10.718517420078616, 0.29188472988065495, -1.2], [-2.310815072326706, 10.718984235455277, 0.5029179530585486, 0.40000000000000013], [-2.250256927274077, 10.7470116403635, 0.6089529669146794, 1.2000000000000006], [-2.4078141528407944, 10.696197951674801, 0.2910470330853207, -1.2], [-2.2625570787999116, 10.786624601979373, 0.5032670160734467, 0.40000000000000013], [-2.37319268235858, 10.803936049039782, 0.3963839209116553, -0.3999999999999999], [-2.4400133449020482, 10.792431192800741, 0.3963141083086757, -0.3999999999999999], [-2.3484550625403937, 10.948347869936686, 0.3954763570729203, -0.3999999999999999], [-2.2532005442925973, 10.986565753726355, 0.6137697234878515, 1.2000000000000006], [-2.2241527610867795, 11.130722431723722, 0.6164922380726879, 1.2000000000000006], [-2.3272220554510197, 11.112000353866012, 0.3944291680282261, -0.3999999999999999], [-2.2968682826047866, 11.131657762965752, 0.5056406445747536, 0.40000000000000013], [-2.2805508875817773, 11.32421563798276, 0.5068972714283867, 0.40000000000000013], [-2.3203488195890745, 11.3333663356091, 0.39296310336565415, -0.3999999999999999], [-2.2253235316083524, 11.390402063747686, 0.6217278430435271, 1.2000000000000006], [-2.23390046248441, 11.420813566670208, 0.5074557722522236, 0.40000000000000013], [-2.315297365324197, 11.574401473618405, 0.391357413497123, -0.3999999999999999], [-2.2168668356954866, 11.63137340411444, 0.6265445996166993, 1.2000000000000006], [-2.3994033185138965, 11.600249851280598, 0.2730365519856337, -1.2], [-2.233080590823236, 11.690844769333019, 0.5092708999296937, 0.40000000000000013], [-2.3589382981537037, 11.726595493110718, 0.27073288579846444, -1.2], [-2.3008663461775223, 11.796656013544418, 0.38989134883455107, -0.3999999999999999], [-2.209460232985442, 11.892117815907735, 0.6317802045875385, 1.2000000000000006], [-2.2516708194251622, 11.903349900014954, 0.3892630354077345, -0.3999999999999999], [-2.324463966690179, 11.881746284197003, 0.26780094701479445, -1.2], [-2.2175289279374653, 11.922764866099948, 0.5108067771952451, 0.40000000000000013], [-2.2538194745555633, 11.911368790129554, 0.2675915228159609, -1.2], [-2.178403555854863, 12.077484518563601, 0.5117841536369597, 0.40000000000000013], [-2.1829008579162608, 12.095192687788384, 0.6357592643653763, 1.2000000000000006], [-2.2383426880850124, 12.155028982889158, 0.3875875329362237, -0.3999999999999999], [-2.2804615843118747, 12.317890670472249, 0.25921455486261813, -1.2], [-2.2227746224162255, 12.415062075134333, 0.2575391612719496, -1.2], [-2.186230627716147, 12.434387153701119, 0.6426702629268841, 1.2000000000000006], [-2.196164124819029, 12.474982005763925, 0.5145068451531648, 0.40000000000000013], [-2.1425536546232067, 12.599100045840768, 0.6458116259093877, 1.2000000000000006], [-2.2643337612516414, 12.581746676789589, 0.3846554036110799, -0.3999999999999999], [-2.198573038349574, 12.65771577116447, 0.2527224046987775, -1.2], [-2.1750587039156537, 12.73714405461915, 0.5162521602276552, 0.40000000000000013], [-2.238686482838199, 12.824800292270476, 0.38304971374254876, -0.3999999999999999], [-2.1747996213790666, 12.920092091405744, 0.24748679972793824, -1.2], [-2.1535345564869504, 13.01725329936264, 0.6543980180615641, 1.2000000000000006], [-2.187058282696622, 13.165406851352257, 0.519184289552799, 0.40000000000000013], [-2.0682676188644926, 13.230434114169201, 0.24162292216059827, -1.2], [-2.249455724453499, 13.24346320074072, 0.3801873970203845, -0.3999999999999999], [-2.168249294443763, 13.280340530506738, 0.2401569527687633, -1.2], [-2.1361605605328022, 13.338559010168616, 0.6608901682254047, 1.2000000000000006], [-2.1577943406236098, 13.438198159944571, 0.520999417230269, 0.40000000000000013], [-2.1011219599138715, 13.601533356858653, 0.6661257731962439, 1.2000000000000006], [-2.2400954133839512, 13.604417430165359, 0.377743955916098, -0.3999999999999999], [-2.1622288912277443, 13.672487145254262, 0.3773948929011999, -0.3999999999999999], [-2.0809447496291567, 13.728170217410458, 0.23136113641775338, -1.2], [-2.148368119037393, 13.828678025980699, 0.5236522961434944, 0.40000000000000013], [-2.1431530665836362, 14.033933863880375, 0.37495145179691336, -0.3999999999999999], [-2.106513383233814, 14.090157922222986, 0.6761781347402553, 1.2000000000000006], [-2.116678410658171, 14.141260966031997, 0.5257466742328829, 0.40000000000000013], [-2.0736923856429295, 14.42245242291376, 0.6828797091029295, 1.2000000000000006], [-2.0946138788714483, 14.532649102029193, 0.5283995531461083, 0.40000000000000013], [-2.152273017194013, 14.572484794069997, 0.3712513838389937, -0.3999999999999999], [-2.0231688076393577, 14.688270075344283, 0.5293769295878229, 0.40000000000000013], [-2.0756120529212976, 14.699000478760663, 0.37048344520621795, -0.3999999999999999], [-2.0476810196035475, 14.823824383301131, 0.6910472528574387, 1.2000000000000006], [8.784462172926562, 11.47924364037722, 0.6985865240154472, 1.2000000000000006], [8.643867253715156, 11.631338367097312, 0.6985865240154472, 1.2000000000000006], [-2.01182307782236, 15.20812065601524, 0.5329373723397832, 0.40000000000000013], [8.86867671544905, 11.41559660678595, 0.6990053724131143, 1.2000000000000006], [8.58702381954077, 11.72028699299172, 0.6990053724131143, 1.2000000000000006], [8.952448256526495, 11.35108640713428, 0.6994242208107815, 1.2000000000000006], [8.751204607664915, 11.589530329880938, 0.699633645009615, 1.2000000000000006], [-2.0698358361213067, 15.238622346987988, 0.36678337724829835, -0.3999999999999999], [8.78228318958885, 11.618259075505645, 0.5334958731636202, 0.40000000000000013], [9.066064089233228, 11.311820599800757, 0.7006807660037829, 1.2000000000000006], [8.586576710391817, 11.864672700124274, 0.7010996144014501, 1.2000000000000006], [8.904607069385332, 11.588375580628155, 0.5339845613844775, 0.40000000000000013], [8.9823118978036, 11.517019884769494, 0.5340543739874571, 0.40000000000000013], [-2.038520846959818, 15.363492520347437, 0.7021467353956179, 1.2000000000000006], [8.791223365347536, 11.769957155305526, 0.5342638117963959, 0.40000000000000013], [8.577157812432615, 12.002632694506751, 0.7029844321909522, 1.2000000000000006], [9.089521761789143, 11.471296644949536, 0.5344034370023552, 0.40000000000000013], [8.747614402156172, 11.874019031613333, 0.5345430622083145, 0.40000000000000013], [9.196614789945517, 11.42431028033962, 0.5347525000172533, 0.40000000000000013], [8.702856524966558, 11.977947480441758, 0.5348223126202329, 0.40000000000000013], [8.551902917074258, 12.126859885849031, 0.7044504015827872, 1.2000000000000006], [9.301763328727434, 11.37452391977877, 0.7052880983781215, 1.2000000000000006], [8.546058430068586, 12.272774370500398, 0.7065446435711229, 1.2000000000000006], [8.713762205484503, 12.13805016075561, 0.5356600638559883, 0.40000000000000013], [9.379898466547676, 11.440670196564861, 0.5357996890619475, 0.40000000000000013], [8.680290014842434, 12.256372289618902, 0.536078939473866, 0.40000000000000013], [-1.9947666269032363, 15.748326418663561, 0.5366374402977029, 0.40000000000000013], [5.4033137061696035, 14.702228724352713, 0.7105237033489606, 1.2000000000000006], [5.31065139179097, 14.760192151279867, 0.5369166907096213, 0.40000000000000013], [5.318145573506214, 14.776082090179019, 0.7111519759454614, 1.2000000000000006], [5.372647557345696, 14.763989846509837, 0.36287387148143985, -0.3999999999999999], [5.430433378499369, 14.758453624273042, 0.5372657537245195, 0.40000000000000013], [5.282599535397169, 14.828571261939807, 0.3627342462754806, -0.3999999999999999], [-2.0630447970868317, 15.828269580660534, 0.3627342462754806, -0.3999999999999999], [-2.0425899368277762, 16.04197255374355, 0.7161781567174671, 1.2000000000000006], [8.986023479525567, 16.697743175440838, 0.7844504455372108, 1.2000000000000006], [8.870510744967275, 16.775657498704163, 0.7844504455372108, 1.2000000000000006], [8.776249405862337, 16.886004939029128, 0.7852881423325451, 1.2000000000000006], [9.255378545456706, 16.596057732863006, 0.7859164149290457, 1.2000000000000006], [9.146441633836046, 16.684541131912827, 0.7861258391278794, 1.2000000000000006], [9.094705994581439, 16.85736482840408, 0.5628171664150587, 0.40000000000000013], [9.445245140600367, 16.620273164434607, 0.7886389295138823, 1.2000000000000006], [8.745638718171325, 17.096618222434593, 0.7886389295138823, 1.2000000000000006], [9.250822015437112, 16.835004830220694, 0.563305854635916, 0.40000000000000013], [8.898582257650931, 17.072593546817984, 0.563305854635916, 0.40000000000000013], [9.372609476756939, 16.761935663932476, 0.5633756672388956, 0.40000000000000013], [9.022240713238299, 17.00273744358763, 0.5633756672388956, 0.40000000000000013], [9.671704217358442, 16.690540187776413, 0.79261798929172, 1.2000000000000006], [8.733353836557999, 17.341528099528503, 0.7928274134905535, 1.2000000000000006], [9.575618663038583, 16.801373411419853, 0.5644228562835899, 0.40000000000000013], [8.86635551362631, 17.284293500790973, 0.5644228562835899, 0.40000000000000013], [-11.730647795102412, 15.437193920648374, 0.09942389115260453, -1.2], [-11.753961919567294, 15.46091854606451, 0.3329242648031848, -0.3999999999999999], [-2.6376199176507695, 22.880864643377365, 0.586553451428128, 0.40000000000000013], [-2.8095170709695823, 22.87690194098971, 0.5866930766340872, 0.40000000000000013], [-2.472177558679492, 22.932903386537202, 0.5867628892370669, 0.40000000000000013], [-2.1457138125258957, 23.092372962417727, 0.5876006404728222, 0.40000000000000013], [-1.975660428365826, 23.120301035359756, 0.5876704530758019, 0.40000000000000013], [-2.830488522803034, 23.021539526550544, 0.8631939442986329, 1.2000000000000006], [-2.321307029798844, 23.112624067398425, 0.5878798908847407, 0.40000000000000013], [-2.664069979468923, 23.075216022238337, 0.8638222168951337, 1.2000000000000006], [-2.4981915740055283, 23.137390254704062, 0.864659913690468, 1.2000000000000006], [-2.3314305321547493, 23.198157106933053, 0.8654976104858023, 1.2000000000000006], [-1.8217528316749911, 23.325992950774253, 0.5889968925324145, 0.40000000000000013], [-2.1768599709453524, 23.37676650480826, 0.8688483976671393, 1.2000000000000006], [-15.001217509405912, 16.7719561296704, 0.31016535623183017, -0.3999999999999999], [-15.131558329077535, 16.65366297795977, 0.31002573102587094, -0.3999999999999999], [-14.921984448489132, 16.935815146369087, 0.30981629321693205, -0.3999999999999999], [-15.241790010790758, 16.749485916960253, 0.026963118356189475, -1.2], [-15.133075455565274, 16.88861418597005, 0.0267536941573559, -1.2], [-15.017973364486107, 17.261437164441947, 0.3077917277305232, -0.3999999999999999], [9.64601974480163, 21.452115753566822, 0.5922780848724565, 0.40000000000000013], [9.496453028675626, 21.54978831901161, 0.8772253656204823, 1.2000000000000006], [9.33857931433906, 21.631972172843444, 0.8772253656204823, 1.2000000000000006], [9.17999443103193, 21.712775206793534, 0.8772253656204823, 1.2000000000000006], [-15.156829567346312, 17.1472706411717, 0.022774634379518044, -1.2], [9.377029264437805, 21.70662736414938, 0.5929762109022526, 0.40000000000000013], [9.544865059367709, 21.641804454240944, 0.5931158361082118, 0.40000000000000013], [9.710389454590258, 21.571913609233842, 0.8797384560064849, 1.2000000000000006], [-1.8772014233671248, 23.929435618135358, 0.8797384560064849, 1.2000000000000006], [9.095883042737146, 21.944626194626313, 0.8807855770006529, 1.2000000000000006], [9.271801932592034, 21.894917952170292, 0.5938139621380081, 0.40000000000000013], [-15.236180272734178, 17.461386956855613, 0.017120181011011648, -1.2], [9.194957789557106, 22.145529906980062, 0.5951404015946207, 0.40000000000000013], [5.3379716006680615, 24.14040468850077, 0.30115953044745974, -0.3999999999999999], [5.346343602955266, 24.94301298686431, 0.29571414741504976, -0.3999999999999999], [-16.03827076279453, 20.400810973707614, 0.28733663505749585, -0.3999999999999999], [-15.917453817284267, 20.56937941691859, 0.2870573846455774, -0.3999999999999999], [-15.794914133758107, 20.737124067829413, 0.28677813423365894, -0.3999999999999999], [-14.857892347507073, 21.847969012040384, 0.2851724443651278, -0.3999999999999999], [-15.023801434595246, 21.725328510394597, 0.2851026317621482, -0.3999999999999999], [-15.339589077483758, 21.460351215716504, 0.2851026317621482, -0.3999999999999999], [-15.650704132941332, 21.189903024072276, 0.2851026317621482, -0.3999999999999999], [-15.201556508849778, 21.61650958244562, 0.28489319395320933, -0.3999999999999999], [-14.728337374906722, 22.016057756865447, 0.2848233813502297, -0.3999999999999999], [-15.626945243640977, 21.4767441096572, 0.28370637970255586, -0.3999999999999999], [9.50763508171292, 26.73975570562619, 0.6252994460818146, 0.40000000000000013], [-1.4252219468434035, 28.59895493907886, 0.6255088838907534, 0.40000000000000013], [9.725543674751258, 26.692789231824694, 0.6255786964937331, 0.40000000000000013], [9.943355423856874, 26.64378657215293, 0.6258579469056516, 0.40000000000000013], [9.334114379546264, 26.89614247546073, 0.6258579469056516, 0.40000000000000013], [9.216574706656742, 27.200382540182076, 0.6275334493771623, 0.40000000000000013], [10.040081267648652, 26.868922071117122, 0.9827751618326013, 1.2000000000000006], [-1.4946609322957394, 29.821814277404098, 1.0022516123241232, 1.2000000000000006], [9.883884675811041, 31.803099088007194, 0.6592981837328874, 0.40000000000000013], [9.665449175747526, 31.97349509801759, 0.659926497159704, 0.40000000000000013], [10.174424429491456, 31.838119222564067, 0.6602057475716224, 0.40000000000000013], [10.17244090528941, 31.83259465007272, 1.0805762626878783, 1.2000000000000006], [-1.0364518801246452, 37.42334336490329, 0.6869439745128152, 0.40000000000000013], [10.026103833352638, 36.8130958059697, 0.6928780457660825, 0.40000000000000013], [9.743408822772697, 36.92812129013003, 0.6930874835750214, 0.40000000000000013], [10.347031193921643, 36.82288619877287, 1.1808904539291583, 1.2000000000000006], [-21.069030510629236, 31.45954783569295, 0.20558607696836614, -0.3999999999999999], [-21.391355310423045, 31.377757000004777, 0.20467851312963112, -0.3999999999999999], [10.4210427571751, 41.72394225688742, 0.7265975330052368, 0.40000000000000013], [10.107451026305094, 41.89078819565647, 0.7271560338290737, 0.40000000000000013], [10.474235594988285, 41.919051326913184, 1.284136583954108, 1.2000000000000006], [10.13857155297352, 42.00899223589921, 1.284136583954108, 1.2000000000000006], [10.830210018606069, 41.90102810572798, 0.7285522858886659, 0.40000000000000013], [-0.709038750028526, 57.66347671663537, 1.5846603092802805, 1.2000000000000006], [11.120605021860856, 56.96437033164037, 0.8312466248716806, 0.40000000000000013], [-0.7151980727209852, 58.133987434462625, 0.8314560626806193, 0.40000000000000013], [1.5195348183779678, 61.52869356204023, 0.04473783970333195, -0.3999999999999999], [5.073212151726797, 61.48708023724171, 0.04362083805565814, -0.3999999999999999], [11.439817695944253, 61.011847285540675, 0.8593811038724656, 0.40000000000000013], [11.689176472740309, 65.06866600393317, 0.8875155828732506, 0.40000000000000013], [14.49832831315618, 65.07219891982305, 1.7750269060199955, 1.2000000000000006], [8.818111571073048, 72.81602044955893, 1.9136657256478184, 1.2000000000000006], [12.551831810983316, 72.91253923612891, 0.9424581014182081, 0.40000000000000013], [13.768405529858791, 72.71844886386302, 1.9283254195661683, 1.2000000000000006], [1.2476421313017925, 74.97736983119862, -0.04909029870127124, -0.3999999999999999], [0.9387629168292289, 75.21210795753403, 0.9506959885698028, 0.40000000000000013], [17.77975821366545, 76.1598746565128, 2.0169118556727685, 1.2000000000000006], [47.35648972259149, 63.571420836353425, 2.052304545275642, 1.2000000000000006], [13.031972557350265, 79.3416128979354, 2.061938058421986, 1.2000000000000006], [24.83184721270082, 81.07466865802802, 2.156178947897092, 1.2000000000000006], [13.551875448365177, 86.71163580640813, 1.0385900557211387, 0.40000000000000013], [52.872675769586, 69.37798867554798, 2.2194250559448303, 1.2000000000000006], [8.915518332671137, 92.0400907270114, 1.0712623539155988, 0.40000000000000013], [9.692181670683942, 91.99867908899289, 1.0715416043275172, 0.40000000000000013], [20.71894414488982, 95.06455786989261, 2.4164932270472192, 1.2000000000000006], [19.150342204408794, 95.56882049865551, 2.4198440142285564, 1.2000000000000006], [23.490178905085354, 95.9928006820069, 2.448953977866423, 1.2000000000000006], [26.036285319817722, 95.81770414584793, 2.4592157636092677, 1.2000000000000006], [14.717578948116746, 99.12164584891, 1.1254369338277803, 0.40000000000000013], [20.65463162219833, 155.2673630873944, 3.658378726130288, 1.2000000000000006], [12.312708261276875, 191.3556263648354, 4.393457664036117, 1.2000000000000006], [14.978259637770336, 232.0240814937235, 2.048848233439155, 0.40000000000000013], [33.73593705129936, 288.53349296533526, 2.4538311433239053, 0.40000000000000013], [8.92096999050232, 17.23708913161584, 0.3356469563193898, -0.3999999999999999], [-2.5256202703736608, 22.68399055587274, 0.31491261323444397, -0.3999999999999999], [-1.8996165215080512, 23.228271875851924, 0.3116314208944021, -0.3999999999999999], [-3.0296332585078587, 23.183843349397314, 0.8671730040764709, 1.2000000000000006], [5.104128617356655, 23.236200962780366, 0.022984058578351618, -1.2], [-1.2548826959515347, 24.01715071826592, 0.01942384719818102, -1.2], [5.221948215230284, 24.444090337557157, -0.0021468452816766903, -1.2], [-2.224688830349968, 25.593404278777417, 0.9151311456093583, 1.2000000000000006], [5.209357772395169, 25.198536731676327, -0.017434811796527283, -1.2], [-1.1725915542855405, 25.874379726198075, -0.019319629586029397, -1.2], [-15.005798944565672, 21.383214801932546, -0.039005504276384995, -1.2], [-14.976356804490646, 21.66777357175441, -0.04319398825305637, -1.2], [-14.955664951264778, 21.9687081224078, -0.04780132062739484, -1.2], [9.275033221452706, 26.45651279141699, 0.277143995022472, -0.3999999999999999], [9.363878146139614, 27.271589550954324, 0.2716287993870824, -0.3999999999999999], [9.371321144452127, 28.564736959442584, 0.26318147442654893, -0.3999999999999999], [10.747513637749273, 30.43885569655537, 1.0575396008161857, 1.2000000000000006], [11.012472531760006, 30.418068389611857, 1.0592149944068543, 1.2000000000000006], [11.266285997376329, 30.367042635463775, 1.060262115401022, 1.2000000000000006], [-20.735017036098906, 31.521767273772653, 0.20663326601306034, -0.3999999999999999], [-20.49557227262787, 31.709735125755284, 0.20656345341008076, -0.3999999999999999], [10.724864676049275, 37.00446773130826, 0.6956007372822874, 0.40000000000000013], [-21.806198041420327, 31.41066071306105, 0.20272376024620187, -0.3999999999999999], [10.97816933233072, 46.72664514439962, 0.7613642092890853, 0.40000000000000013], [-33.95444016665767, 37.454440166657676, 0.11475988049188635, -0.3999999999999999], [-33.46782468155926, 38.15694699438283, 0.11364287884421248, -0.3999999999999999], [-32.258000408687934, 39.32613895725404, 0.11343344103527364, -0.3999999999999999], [-34.39923085728631, 37.30403001674005, 0.11329381582931441, -0.3999999999999999], [11.618566184124763, 57.01187131155995, 0.8322938139163747, 0.40000000000000013], [16.615400312068406, 60.50485600252477, 1.6937703168725702, 1.2000000000000006], [13.205163345895427, 64.3192947748755, 1.7536656377389712, 1.2000000000000006], [20.538690765112868, 64.00503191176435, 1.7884300547453438, 1.2000000000000006], [13.026046392769018, 79.30712465157343, 0.9869985421192027, 0.40000000000000013], [27.29899080749756, 81.67230442986731, 2.1844512147396244, 1.2000000000000006], [33.69042505267091, 80.06731529671714, 2.2022522716404778, 1.2000000000000006], [29.157427120978678, 82.5346645544511, 2.2146082993716583, 1.2000000000000006], [27.17382907061827, 93.78874887901951, 2.425079619199396, 1.2000000000000006], [34.761055666251615, 92.88790635480824, 2.4590063394104344, 1.2000000000000006], [-2.729118001525531, 22.918683596868465, 0.31309748555697403, -0.3999999999999999], [9.124522914489708, 21.80096170236561, 0.3072332269066863, -0.3999999999999999], [-1.5170192378515415, 28.303045293335575, 0.2765156815956554, -0.3999999999999999], [-1.3900091234452605, 30.022954081648294, 0.2645777264861412, -0.3999999999999999], [4.034616118215339, 61.19769858054814, 0.04620390436590388, -0.3999999999999999], [26.121526235859253, 82.71602090547535, 2.197226090868472, 1.2000000000000006]]
  in  "lane width":dbl=3.5
  out "XY Graph":cluster{"Y":dbl[], "Y":dbl[]}[](graph)
  out "seed_y":dbl[](array[numeric])
  out "seed_x":dbl[](array[numeric])
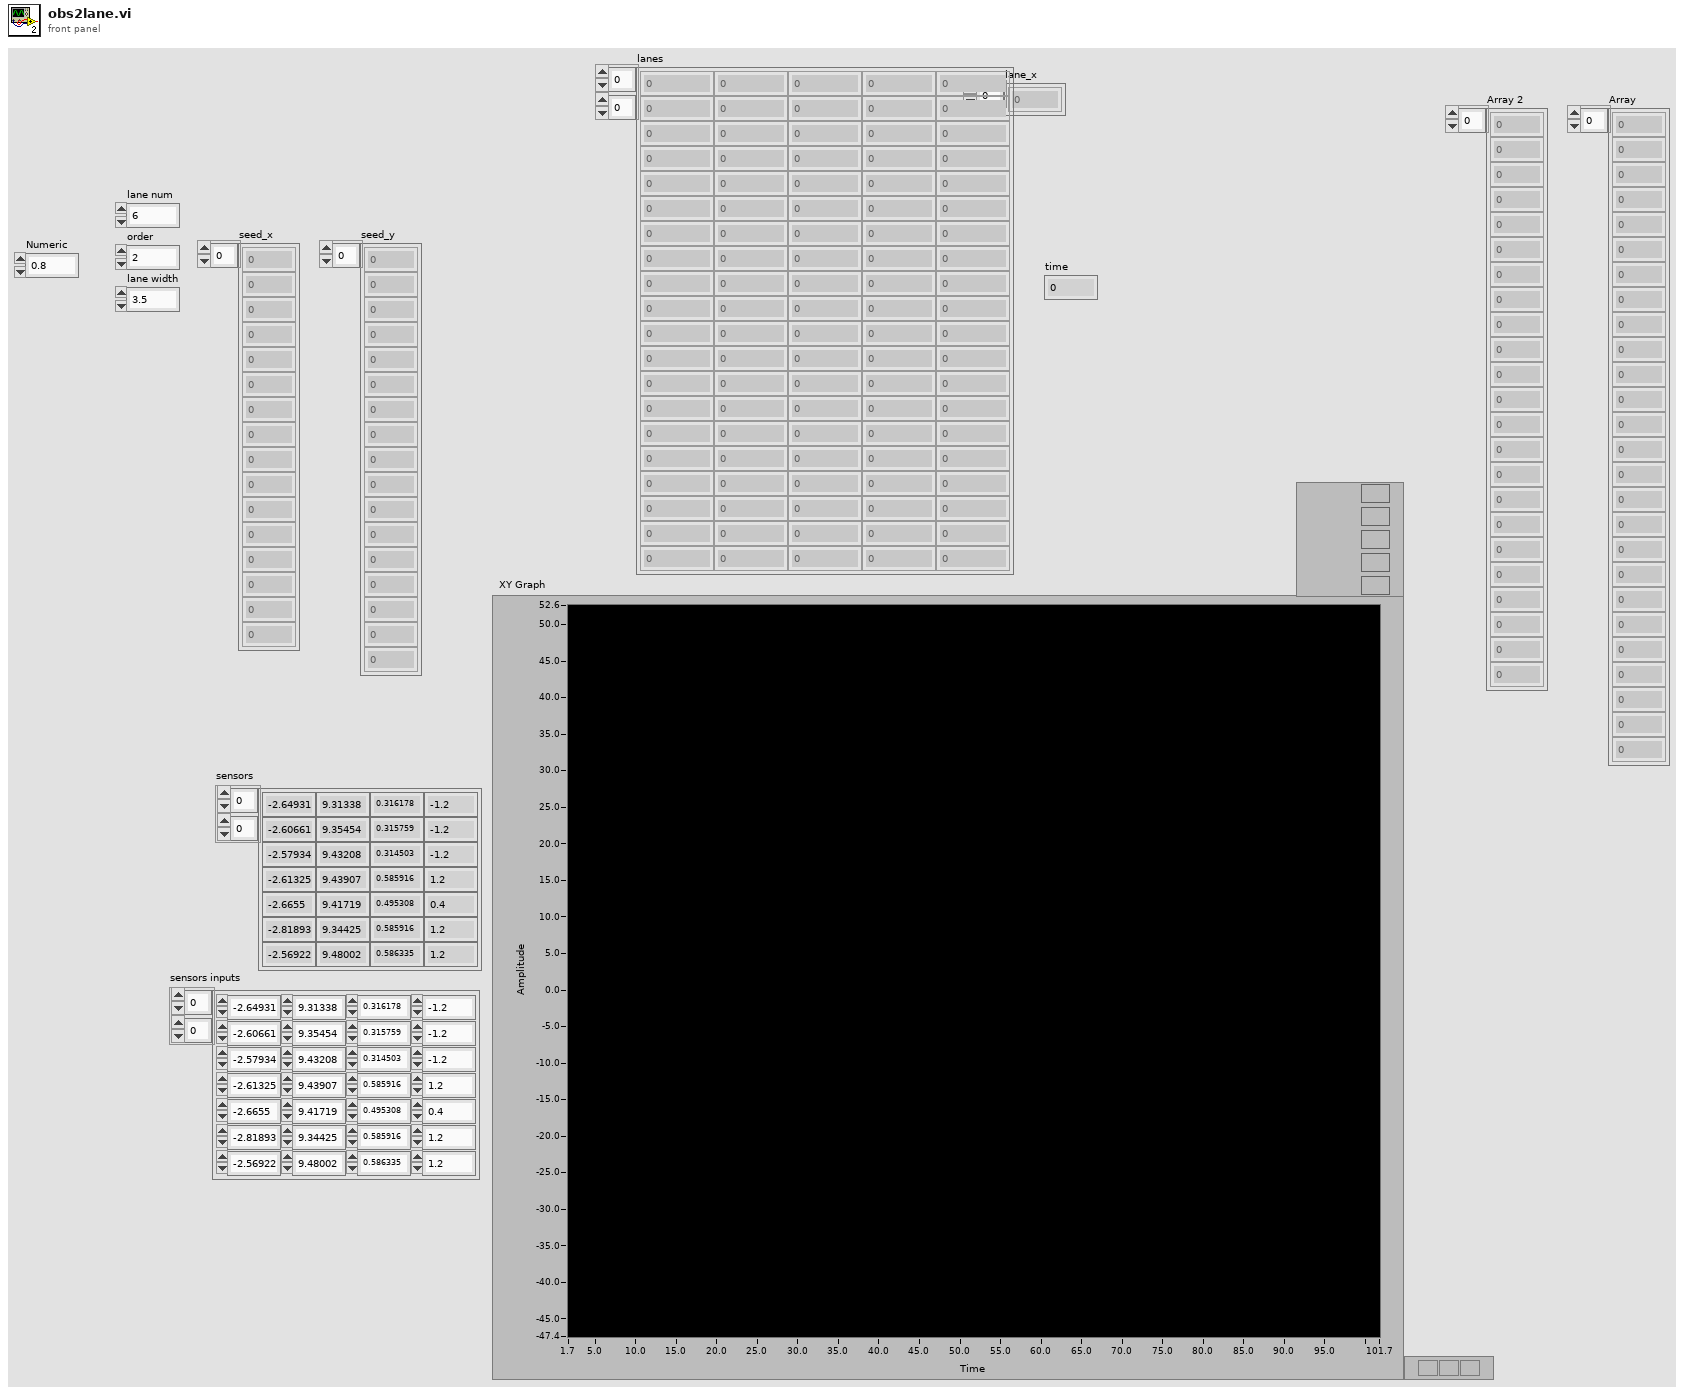
[diagram p1: front panel]
types:
  T1 = typedef "NI_Matrix.lvlib/RealMatrix.ctl" = dbl[][]
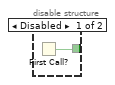
[diagram p3: hidden frame]
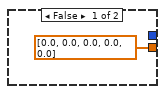
[diagram p5: hidden frame]
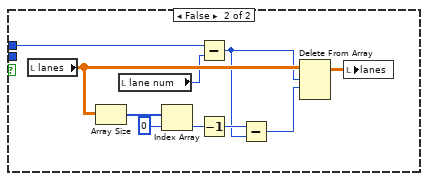
[diagram p12: hidden frame]
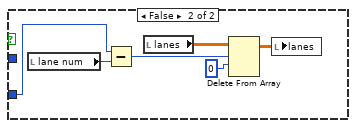
[diagram p14: hidden frame]
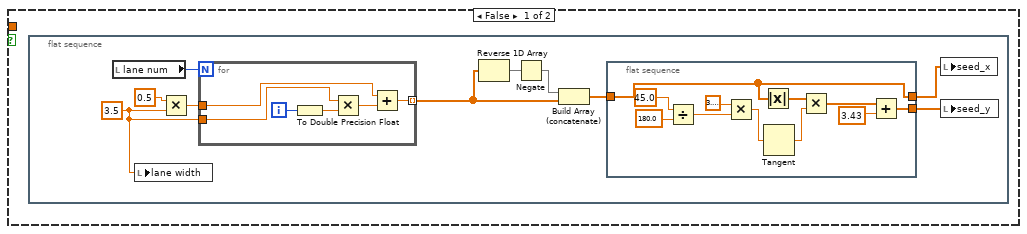
[diagram p15: hidden frame]
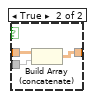
[diagram p16: hidden frame]
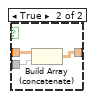
[diagram p17: hidden frame]
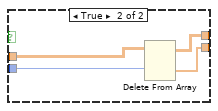
[diagram p18: hidden frame]
diagram:
  n1 = flat-sequence {
    tunnel: [w3] -> w2
    tunnel: w2 -> [w5]
    tunnel: [w5] -> w1
    tunnel: w1 -> [w616]
    frame #0 {
      n2 = Tick Count (ms)() -> (millisecond timer value=w3:u32)
    }
    frame #1 {
      n3 = flat-sequence {
        tunnel: [w68] -> w4
        tunnel: w4 -> [w85]
        frame #0 {
          n4 = disable-structure shown="Enabled" {
            disable-tunnel: [w9 _] -> w6
            frame Enabled {
              n5 = global read "G_SEN.vi" "sensor_velodyne_chopped"() -> (w8:dbl[][])
              n6 = global read "G_SEN.vi" "sensor_lane"() -> (w10:dbl[][])
              n7 = global read "G_SEN.vi" "sensor_obs"() -> (w11:dbl[][])
              n8 = Build Array (concatenate)(w11, w10, w8, "sensors inputs") -> (w9:dbl[][])
            }
            frame Disabled {
            }
          }
          "sensors" <- w6
        }
        frame #1 {
          n9 = disable-structure shown="Enabled" {
            disable-tunnel: [w13 _] -> w12
            frame Disabled {
              n10 = First Call?() -> (First Call?: T/F=w13:bool)
            }
            frame Enabled {
            }
          }
          n11 = case shown="True" w12 {
            frame False {
            }
            frame True {
              n12 = local read "lane width"() -> (w19:dbl)
              n13 = local write "lane width"(3.5 ("lane width")) -> ()
              n14 = for {
                N: 1000 -> [_]
                tunnel: [w38] -> w17 mode=indexing
                i -> [w41]
                n15 = To Double Precision Float(number=w41) -> (double precision float=w40:dbl)
                n16 = Multiply(x=0.1, y=w40) -> (x*y=w38:dbl)
              }
              "lane_x" <- w17
              n17 = local read "lane num"() -> (w15:i32)
              n18 = Multiply(x=0.5, y=w19) -> (x*y=w25:dbl)
              n19 = for {
                N: w15 -> [_]
                tunnel: w19 -> [w47]
                tunnel: w25 -> [w43]
                tunnel: [w42] -> w22 mode=indexing
                i -> [w46]
                n20 = To Double Precision Float(number=w46) -> (double precision float=w45:dbl)
                n21 = Multiply(x=w47, y=w45) -> (x*y=w44:dbl)
                n22 = Add(x=w43, y=w44) -> (x+y=w42:dbl)
              }
              n23 = Reverse 1D Array(array=w22) -> (reversed array=w24:dbl[])
              n24 = Negate(x=w24) -> (-x=w23:dbl[])
              n25 = Build Array (concatenate)(w23, w22) -> (w20:dbl[])
              n26 = flat-sequence {
                tunnel: [w29] -> w21
                tunnel: w20 -> [w27]
                tunnel: [w27] -> w16
                frame #0 {
                  n27 = Divide(x=45.0, y=180.0) -> (x/y=w34:dbl)
                  n28 = Multiply(x=3.141592653589793, y=w34) -> (x*y=w33:dbl)
                  n29 = Absolute Value(x=w27) -> (abs(x)=w28:dbl[])
                  n30 = Tangent(1:w33) -> (0:w32:dbl)
                  n31 = Multiply(x=w28, y=w32) -> (x*y=w31:dbl[])
                  n32 = Add(x=w31, y=3.43) -> (x+y=w29:dbl[])
                }
              }
              "seed_x" <- w16
              "seed_y" <- w21
            }
          }
        }
        frame #2 {
          n33 = local read "sensors"() -> (w49:dbl[][])
          n34 = local read "sensors"() -> (w48:dbl[][])
          n35 = Index Array(array=w49, index (col)=0 ("disabled index (col)")) -> (element=w66:dbl[])  [unwired: 1 in]
          n36 = Index Array(array=w48, index (col)=1 ("disabled index (col)")) -> (element=w64:dbl[])  [unwired: 1 in]
          n37 = local read "seed_x"() -> (w70:dbl[])
          n38 = local read "seed_y"() -> (w69:dbl[])
          n39 = for {
            tunnel: w70 -> [w82] mode=indexing
            tunnel: w66 -> [w83]
            tunnel: [w80] -> w58 mode=indexing
            tunnel: w69 -> [w79] mode=indexing
            tunnel: w64 -> [w78]
            tunnel: [w77] -> w63 mode=indexing
            n40 = Subtract(x=w83, y=w82) -> (x-y=w81:dbl[])
            n41 = Subtract(x=w79, y=w78) -> (x-y=w73:dbl[])
            n42 = Multiply(x=w73, y=0.25) -> (x*y=w71:dbl[])
            n43 = Square(x=w81) -> (x^2=w76:dbl[])
            n44 = Square(x=w71) -> (x^2=w74:dbl[])
            n45 = Add(x=w76, y=w74) -> (x+y=w75:dbl[])
            n46 = Array Max & Min(array=w75) -> (min value=w77:dbl, min index (indices)=w80:i32)  [unwired: 2 out]
          }
          n47 = local read "lane width"() -> (w61:dbl)
          n48 = Square Root(x=w63) -> (sqrt(x)=w50:dbl[])
          n49 = Multiply(x=0.8, y=w61) -> (x*y=w51:dbl)
          n50 = Greater?(x=w51, y=w50) -> (0:w57:bool[])
          n51 = Not(x=w57) -> (.not. x?=w56:bool[])
          n52 = Boolean To (0,1)(Boolean=w57) -> (0, 1=w60:i16[])
          n53 = Boolean To (0,1)(Boolean=w56) -> (0, 1=w55:i16[])
          n54 = To Long Integer(number=w60) -> (32bit integer=w59:i32[])
          n55 = To Long Integer(number=w55) -> (32bit integer=w54:i32[])
          n56 = Multiply(x=w59, y=w58) -> (x*y=w52:i32[])
          n57 = Negate(x=w54) -> (-x=w53:i32[])
          n58 = Add(x=w53, y=w52) -> (x+y=w68:i32[])
        }
        frame #3 {
          n59 = local read "lane width"() -> (w91:dbl)
          n60 = local read "sensors"() -> (w89:dbl[][])
          n61 = Index Array(array=w89, index (col)=1 ("disabled index (col)")) -> (element=w94:dbl[])  [unwired: 1 in]
          n62 = Multiply(x=w91, y=0.01) -> (x*y=w93:dbl)
          n63 = Multiply(x=w93, y=w94) -> (x*y=w96:dbl[])
          n64 = Max & Min(x=0.3 ("y"), y=w96) -> (max(x,y)=w88:dbl[])  [unwired: 1 out]
          n65 = for {
            tunnel: w85 -> [w102] mode=indexing
            tunnel: w88 -> [w101]
            tunnel: [w100] -> w87 mode=indexing
            tunnel: [w99] -> w86 mode=indexing
            tunnel: [w97] -> w84 mode=indexing
            i -> [w98]
            n66 = Greater Or Equal To 0?(x=w102) -> (x >= 0?=w103:bool)
            n67 = case shown="True" w103 {
              tunnel: w102 -> [_ w123]
              tunnel: w101 -> [_ w124]
              tunnel: [dbl[] [0.0, 0.0, 0.0, 0.0, 0.0] w108] -> w100
              tunnel: [_ w107] -> w99
              tunnel: w98 -> [_ _]
              tunnel: [_ w105] -> w97
              frame False {
              }
              frame True {
                n68 = local read "sensors"() -> (w122:dbl[][])
                n69 = Index Array(array=w122, index (col) #1=1 ("disabled index (col)"), index (col) #2=0 ("disabled index (col)")) -> (element #1=w114:dbl[], element #2=w119:dbl[])  [unwired: 2 in]
                n70 = Index Array(array=w119, index=w123) -> (element=w117:dbl)
                n71 = Subtract(x=w119, y=w117) -> (x-y=w120:dbl[])
                n72 = Absolute Value(x=w120) -> (abs(x)=w118:dbl[])
                n73 = Less?(x=w118, y=w124) -> (x < y?=w112:bool[])
                n74 = Greater?(x=100.0 ("y"), y=w114) -> (0:w113:bool[])
                n75 = And(x=w113, y=w112) -> (x .and. y?=w111:bool[])
                n76 = for {
                  N: 3 -> [_]
                  tunnel: [w134] -> w109
                  shift-right: [w132] -> _
                  shift-left: w111 -> [w133]
                  tunnel: [w131] -> w107
                  tunnel: [w130] -> w106
                  tunnel: [w129] -> w105
                  stop <- w130 stop-if-true
                  n77 = flat-sequence {
                    tunnel: [w161] -> w134
                    tunnel: w133 -> [w166]
                    tunnel: [w167] -> w132
                    frame #0 {
                      n78 = local read "sensors"() -> (w171:dbl[][])
                      n79 = local read "sensors"() -> (w180:dbl[][])
                      n80 = Boolean To (0,1)(Boolean=w166) -> (0, 1=w184:i16[])
                      n81 = To Double Precision Float(number=w184) -> (double precision float=w177:dbl[])
                      n82 = Index Array(array=w171, index (col)=1 ("disabled index (col)")) -> (element=w170:dbl[])  [unwired: 1 in]
                      n83 = Index Array(array=w180, index (col)=0 ("disabled index (col)")) -> (element=w176:dbl[])  [unwired: 1 in]
                      n84 = Multiply(x=w170, y=w177) -> (x*y=w174:dbl[])
                      n85 = Negate(x=w176) -> (-x=w173:dbl[])
                      n86 = Multiply(x=w177, y=w173) -> (x*y=w175:dbl[])
                      n87 = flat-sequence {
                        tunnel: [w234] -> w183
                        tunnel: w177 -> [w233]
                        tunnel: w174 -> [w232]
                        frame #0 {
                          n88 = Multiply(x=w232, y=w232) -> (x*y=w224:dbl[])
                          n89 = Add Array Elements(numeric array=w233) -> (sum=w220:dbl)
                          n90 = Multiply(x=w232, y=w224) -> (x*y=w228:dbl[])
                          n91 = Add Array Elements(numeric array=w224) -> (sum=w230:dbl)
                          n92 = Multiply(x=w232, y=w228) -> (x*y=w226:dbl[])
                          n93 = Add Array Elements(numeric array=w228) -> (sum=w229:dbl)
                          n94 = Multiply(x=w232, y=w226) -> (x*y=w222:dbl[])
                          n95 = Add Array Elements(numeric array=w226) -> (sum=w227:dbl)
                          n96 = Multiply(x=w232, y=w222) -> (x*y=w223:dbl[])
                          n97 = Add Array Elements(numeric array=w222) -> (sum=w225:dbl)
                          n98 = Add Array Elements(numeric array=w223) -> (sum=w221:dbl)
                          n99 = Add Array Elements(numeric array=w232) -> (sum=w231:dbl)
                          n100 = Build Array(w221, w225, w227, w229, w230, w231, w220) -> (w234:dbl[])
                        }
                      }
                      n101 = flat-sequence {
                        tunnel: w174 -> [w219]
                        tunnel: w175 -> [w217]
                        tunnel: [w210] -> w163
                        frame #0 {
                          n102 = Multiply(x=w219, y=w217) -> (x*y=w215:dbl[])
                          n103 = Add Array Elements(numeric array=w217) -> (sum=w218:dbl)
                          n104 = Multiply(x=w219, y=w215) -> (x*y=w212:dbl[])
                          n105 = Add Array Elements(numeric array=w215) -> (sum=w216:dbl)
                          n106 = Multiply(x=w219, y=w212) -> (x*y=w213:dbl[])
                          n107 = Add Array Elements(numeric array=w212) -> (sum=w214:dbl)
                          n108 = Add Array Elements(numeric array=w213) -> (sum=w211:dbl)
                          n109 = Build Array(w211, w214, w216, w218) -> (w210:dbl[])
                        }
                      }
                      n110 = for {
                        N: 4 -> [_]
                        tunnel: w183 -> [w238]
                        tunnel: [w235] -> w165 mode=indexing
                        i -> [w237]
                        n111 = Array Subset(array=w238, index=w237, length=4) -> (w235:dbl[])
                      }
                      n112 = local read "order"() -> (w159:i32)
                      n113 = Array Subset(array=w165, index (row)=w159, index (col)=w159) -> (w164:dbl[][])  [unwired: 2 in]
                      n114 = local read "order"() -> (w160:i32)
                      n115 = call-poly <vilib>:"Array To Matrix.vi"("Real 2D Array"=w164) -> ("Real Matrix"=w179:T1)
                      n116 = local read "order"() -> (w157:i32)
                      n117 = Array Subset(array=w163, index=w160) -> (w162:dbl[])  [unwired: 1 in]
                      n118 = call-poly <vilib>:"Inverse Matrix.vi"("Input Matrix"=w179) -> ("Inverse Matrix"=w178:T1)  [unwired: 1 in, 1 out]
                      n119 = Array Subset(array=dbl[] [0.0, 0.0], index=0, length=w157) -> (w155:dbl[])
                      n120 = call-poly <vilib>:"A x B.vi"("Vector"=w162, "A"=w178) -> ("A x Vector"=w169:dbl[])  [unwired: 1 out]
                      n121 = Build Array (concatenate)(w155, w169, 1.0) -> (w161:dbl[])
                      n122 = flat-sequence {
                        tunnel: w161 -> [w199]
                        tunnel: [w187] -> w167
                        tunnel: w166 -> [w186]
                        frame #0 {
                          n123 = local read "sensors"() -> (w193:dbl[][])
                          n124 = Index Array(array=w193, index (col)=1 ("disabled index (col)")) -> (element=w192:dbl[])  [unwired: 1 in]
                          n125 = Multiply(x=w192, y=w192) -> (x*y=w201:dbl[])
                          n126 = local read "sensors"() -> (w190:dbl[][])
                          n127 = Multiply(x=w192, y=w201) -> (x*y=w202:dbl[])
                          n128 = Index Array(array=w199, index #1=0 ("index")) -> (element #1=w203:dbl, element #2=w204:dbl, element #3=w205:dbl, element #4=w209:dbl)  [unwired: 3 in]
                          n129 = Multiply(x=w202, y=w203) -> (x*y=w206:dbl[])
                          n130 = Multiply(x=w201, y=w204) -> (x*y=w207:dbl[])
                          n131 = Multiply(x=w192, y=w205) -> (x*y=w208:dbl[])
                          n132 = Index Array(array=w190, index (col)=0 ("disabled index (col)")) -> (element=w191:dbl[])  [unwired: 1 in]
                          n133 = Negate(x=w191) -> (-x=w188:dbl[])
                          n134 = Compound Arithmetic op=ADD(w206, w207, w208, w209) -> (w198:dbl[])
                          n135 = Subtract(x=w198, y=w188) -> (x-y=w197:dbl[])
                          n136 = Absolute Value(x=w197) -> (abs(x)=w196:dbl[])
                          n137 = Less?(x=w196, y=0.5) -> (x < y?=w185:bool[])
                          n138 = And(x=w186, y=w185) -> (x .and. y?=w187:bool[])
                        }
                      }
                    }
                  }
                  n139 = flat-sequence {
                    tunnel: w132 -> [w149]
                    tunnel: [w153] -> w131
                    tunnel: [w136] -> w130
                    tunnel: [w135] -> w129
                    frame #0 {
                      n140 = local read "sensors"() -> (w152:dbl[][])
                      n141 = Not(x=w149) -> (.not. x?=w148:bool[])
                      n142 = Boolean To (0,1)(Boolean=w148) -> (0, 1=w147:i16[])
                      n143 = Boolean To (0,1)(Boolean=w149) -> (0, 1=w150:i16[])
                      n144 = Index Array(array=w152, index (col)=1 ("disabled index (col)")) -> (element=w146:dbl[])  [unwired: 1 in]
                      n145 = Add Array Elements(numeric array=w150) -> (sum=w153:i16)
                      n146 = Multiply(x=w146, y=w150) -> (x*y=w143:dbl[])
                      n147 = Multiply(x=999.0, y=w147) -> (x*y=w144:dbl[])
                      n148 = Add(x=w143, y=w144) -> (x+y=w142:dbl[])
                      n149 = Array Max & Min(array=w143) -> (max value=w140:dbl)  [unwired: 3 out]
                      n150 = Array Max & Min(array=w142) -> (min value=w141:dbl)  [unwired: 3 out]
                      n151 = Subtract(x=w140, y=w141) -> (x-y=w135:dbl)
                      n152 = Less?(x=w153, y=i16 40) -> (x < y?=w138:bool)
                      n153 = Less?(x=w135, y=14.0) -> (x < y?=w137:bool)
                      n154 = Or(x=w138, y=w137) -> (x .or. y?=w136:bool)
                    }
                  }
                }
                n155 = flat-sequence {
                  tunnel: w109 -> [w127]
                  tunnel: [w126] -> w108
                  tunnel: w106 -> [w125]
                  frame #0 {
                    n156 = Select(t=dbl[] [0.0, 0.0, 0.0, 0.0, 0.0], s=w125, f=w127) -> (s? t:f=w126:dbl[])
                  }
                }
              }
            }
          }
          "lanes" <- w87
          "Array 2" <- w86
          "Array" <- w84
        }
        frame #4 {
          n157 = local read "lanes"() -> (w245:dbl[][])
          n158 = Index Array(array=w245, index (col)=4 ("disabled index (col)")) -> (element=w242:dbl[])  [unwired: 1 in]
          n159 = Array Size(array=w242) -> (size(s)=w241:i32)
          n160 = for {
            N: w241 -> [_]
            shift-right: [w259] -> w240
            shift-left: dbl[][] [] -> [w258]
            shift-right: [w254] -> _
            shift-left: w242 -> [w255]
            i -> [w257]
            n161 = Index Array(array=w255, index=w257) -> (element=w256:dbl)
            n162 = Not Equal To 0?(x=w256) -> (x != 0?=w260:bool)
            n163 = case shown="True" w260 {
              tunnel: w257 -> [_ w278]
              tunnel: [w262 w277] -> w259
              tunnel: w258 -> [w262 w276]
              tunnel: w255 -> [w261 w274]
              tunnel: [w261 w273] -> w254
              frame False {
              }
              frame True {
                n164 = local read "lanes"() -> (w272:dbl[][])
                n165 = Index Array(array=w272, index (col)=3 ("disabled index (col)")) -> (element=w263:dbl[])  [unwired: 1 in]
                n166 = Index Array(array=w263, index=w278) -> (element=w264:dbl)
                n167 = Equal?(x=w264, y=w263) -> (x = y?=w270:bool[])
                n168 = Boolean To (0,1)(Boolean=w270) -> (0, 1=w275:i16[])
                n169 = To Double Precision Float(number=w275) -> (double precision float=w266:dbl[])
                n170 = Array Max & Min(array=w275) -> (max index (indices)=w268:i32)  [unwired: 3 out]
                n171 = local read "lanes"() -> (w269:dbl[][])
                n172 = Subtract(x=w274, y=w266) -> (x-y=w265:dbl[])
                n173 = Replace Array Subset(array=w274, new element=w265) -> (w273:dbl[])  [unwired: 1 in]
                n174 = Index Array(array=w269, index (row)=w268) -> (element=w267:dbl[])  [unwired: 1 in]
                n175 = Build Array (concatenate)(w276, w267) -> (w277:dbl[][])
              }
            }
          }
          n176 = Array Subset(array=w240, index (row)=1 ("index")) -> (w247:dbl[][])  [unwired: 3 in]
          n177 = Array Size(array=w247) -> (size(s)=w252:i32[])
          n178 = Index Array(array=w252, index=0) -> (element=w239:i32)
          n179 = Array Subset(array=w240, index (row)=0 ("index"), length (row)=1 ("length")) -> (w248:dbl[][])  [unwired: 2 in]
          n180 = for {
            N: w239 -> [_]
            shift-right: [w279] -> w246
            shift-left: w248 -> [w282]
            tunnel: w247 -> [w280] mode=indexing
            n181 = Array Size(array=w282) -> (size(s)=w294:i32[])
            n182 = Index Array(array=w280, index=3) -> (element=w288:dbl)
            n183 = Index Array(array=w294, index=0) -> (element=w293:i32)
            n184 = Decrement(x=w293) -> (x-1=w292:i32)
            n185 = Index Array(array=w282, index (row)=w292, index (col)=3 ("disabled index (col)")) -> (element=w289:dbl)
            n186 = local read "lane width"() -> (w286:dbl)
            n187 = Subtract(x=w289, y=w288) -> (x-y=w287:dbl)
            n188 = Divide(x=w287, y=w286) -> (x/y=w285:dbl)
            n189 = Round To Nearest(number=w285) -> (nearest integer value=w284:dbl)
            n190 = Decrement(x=w284) -> (x-1=w283:dbl)
            n191 = for {
              N: w283 -> [_]
              shift-right: [w297] -> w281
              shift-left: w282 -> [w298]
              n192 = Build Array (concatenate)(w298, dbl[] [0.0, 0.0, 0.0, 0.0, 0.0]) -> (w297:dbl[][])
            }
            n193 = Build Array (concatenate)(w281, w280) -> (w279:dbl[][])
          }
          n194 = local write "lanes"(w246) -> ()
        }
        frame #5 {
          n195 = local read "lanes"() -> (w301:dbl[][])
          n196 = Index Array(array=w301, index (col)=4 ("disabled index (col)")) -> (element=w299:dbl[])  [unwired: 1 in]
          n197 = for {
            tunnel: w299 -> [w305] mode=indexing
            tunnel: w299 -> [w302]
            i -> [w303]
            n198 = Equal To 0?(x=w305) -> (x = 0?=w304:bool)
            n199 = case shown="True" w304 {
              tunnel: w303 -> [_ w307]
              tunnel: w302 -> [_ w306]
              frame False {
              }
              frame True {
                n200 = Array Subset(array=w306, index=0, length=w307) -> (w319:dbl[])
                n201 = Increment(x=w307) -> (x+1=w313:i32)
                n202 = Reverse 1D Array(array=w319) -> (reversed array=w312:dbl[])
                n203 = Array Subset(array=w306, index=w313) -> (w321:dbl[])  [unwired: 1 in]
                n204 = Array Size(array=w312) -> (size(s)=w311:i32)
                n205 = Array Max & Min(array=w312) -> (max value=w318:dbl, max index (indices)=w310:i32)  [unwired: 2 out]
                n206 = Array Max & Min(array=w321) -> (max value=w320:dbl, max index (indices)=w314:i32)  [unwired: 2 out]
                n207 = Subtract(x=w311, y=w310) -> (x-y=w309:i32)
                n208 = Not Equal To 0?(x=w318) -> (x != 0?=w317:bool)
                n209 = Not Equal To 0?(x=w320) -> (x != 0?=w316:bool)
                n210 = Decrement(x=w309) -> (x-1=w308:i32)
                n211 = And(x=w317, y=w316) -> (x .and. y?=w315:bool)
                n212 = case shown="True" w315 {
                  tunnel: w314 -> [_ w342]
                  tunnel: w313 -> [_ w341]
                  tunnel: w308 -> [_ w340]
                  tunnel: w307 -> [_ w339]
                  frame False {
                  }
                  frame True {
                    n213 = Add(x=w342, y=w341) -> (x+y=w333:i32)
                    n214 = local read "lanes"() -> (w325:dbl[][])
                    n215 = Subtract(x=w340, y=w339) -> (x-y=w338:i32)
                    n216 = Subtract(x=w339, y=w333) -> (x-y=w337:i32)
                    n217 = Subtract(x=w340, y=w333) -> (x-y=w336:i32)
                    n218 = Divide(x=w338, y=w336) -> (x/y=w331:dbl)
                    n219 = Divide(x=w337, y=w336) -> (x/y=w334:dbl)
                    n220 = Index Array(array=w325, index (row) #1=w340, index (row) #2=w333) -> (element #1=w335:dbl[], element #2=w332:dbl[])  [unwired: 2 in]
                    n221 = Multiply(x=w335, y=w334) -> (x*y=w330:dbl[])
                    n222 = Multiply(x=w332, y=w331) -> (x*y=w329:dbl[])
                    n223 = Add(x=w330, y=w329) -> (x+y=w328:dbl[])
                    n224 = Replace Array Subset(array=w328, new element=0.0 ("new element/subarray"), index=4) -> (w323:dbl[])
                    n225 = Replace Array Subset(array=w325, new element=w323, index (row)=w339) -> (w324:dbl[][])  [unwired: 1 in]
                    n226 = local write "lanes"(w324) -> ()
                  }
                }
              }
            }
          }
        }
        frame #6 {
          n227 = for {
            N: 2 -> [_]
            n228 = flat-sequence {
              tunnel: [w349] -> w347
              tunnel: [w348] -> w346
              tunnel: w347 -> [w372]
              tunnel: [w374] -> w345
              tunnel: w346 -> [w374]
              tunnel: [w372] -> w344
              tunnel: w345 -> [w418]
              tunnel: w344 -> [w420]
              frame #0 {
                n229 = local read "lanes"() -> (w355:dbl[][])
                n230 = Index Array(array=w355, index (col)=3 ("disabled index (col)")) -> (element=w353:dbl[])  [unwired: 1 in]
                n231 = Array Size(array=w353) -> (size(s)=w352:i32)
                n232 = Greater?(x=w352, y=1) -> (0:w350:bool)
                n233 = case shown="True" w350 {
                  tunnel: w353 -> [_ w358]
                  tunnel: [_ w357] -> w349
                  tunnel: [_ w356] -> w348
                  frame False {
                  }
                  frame True {
                    n234 = Less Than 0?(x=w358) -> (x < 0?=w369:bool[])
                    n235 = Boolean To (0,1)(Boolean=w369) -> (0, 1=w368:i16[])
                    n236 = Array Size(array=w368) -> (size(s)=w367:i32)
                    n237 = Array Max & Min(array=w368) -> (max index (indices)=w356:i32)  [unwired: 3 out]
                    n238 = Subtract(x=w367, y=w356) -> (x-y=w357:i32)
                    n239 = Decrement(x=w356) -> (x-1=w366:i32)
                    n240 = Index Array(array=w358, index #1=w366, index #2=w356) -> (element #1=w365:dbl, element #2=w364:dbl)
                    n241 = Subtract(x=w365, y=w364) -> (x-y=w363:dbl)
                    n242 = In Range and Coerce(upper limit=4.0, x=w363, lower limit=3.0) -> (coerced(x)=w359:dbl, In Range?=w360:bool)
                    n243 = case shown="True" w360 {
                      tunnel: w359 -> [_ w370]
                      frame False {
                      }
                      frame True {
                        n244 = local write "lane width"(w370) -> ()
                      }
                    }
                  }
                }
              }
              frame #1 {
                n245 = local read "lane num"() -> (w371:i32)
                n246 = Less Or Equal?(x=w372, y=w371) -> (x <= y?=w373:bool)
                n247 = case shown="True" w373 {
                  tunnel: w374 -> [w381 _]
                  tunnel: w372 -> [w375 w408]
                  frame True {
                    n248 = Equal To 0?(x=w375) -> (x = 0?=w380:bool)
                    n249 = Not Equal To 0?(x=w381) -> (x != 0?=w379:bool)
                    n250 = Not Equal To 0?(x=w375) -> (x != 0?=w377:bool)
                    n251 = And(x=w380, y=w379) -> (x .and. y?=w378:bool)
                    n252 = Or(x=w377, y=w378) -> (x .or. y?=w376:bool)
                    n253 = case shown="True" w376 {
                      tunnel: w375 -> [_ w383]
                      frame False {
                      }
                      frame True {
                        n254 = local read "lanes"() -> (w386:dbl[][])
                        n255 = local read "lane num"() -> (w382:i32)
                        n256 = Array Size(array=w386) -> (size(s)=w394:i32[])
                        n257 = Subtract(x=w382, y=w383) -> (x-y=w392:i32)
                        n258 = Index Array(array=w394, index=0) -> (element=w385:i32)
                        n259 = Decrement(x=w385) -> (x-1=w384:i32)
                        n260 = Index Array(array=w386, index (row)=w384) -> (element=w391:dbl[])  [unwired: 1 in]
                        n261 = Index Array(array=w391, index=3) -> (element=w389:dbl)
                        n262 = for {
                          N: w392 -> [_]
                          tunnel: w391 -> [w406]
                          tunnel: w389 -> [w400]
                          tunnel: [w397] -> w387 mode=indexing
                          i -> [w405]
                          n263 = local read "lane width"() -> (w403:dbl)
                          n264 = Increment(x=w405) -> (x+1=w404:i32)
                          n265 = To Double Precision Float(number=w404) -> (double precision float=w402:dbl)
                          n266 = Multiply(x=w403, y=w402) -> (x*y=w401:dbl)
                          n267 = Subtract(x=w400, y=w401) -> (x-y=w399:dbl)
                          n268 = Replace Array Subset(array=w406, new element #1=w399, index #1=3 ("index"), new element #2=0.0 ("new element/subarray"), index #2=4 ("index")) -> (w397:dbl[])
                        }
                        n269 = Build Array (concatenate)(w386, w387) -> (w388:dbl[][])
                        n270 = local write "lanes"(w388) -> ()
                      }
                    }
                  }
                  frame False {
                    n271 = local read "lanes"() -> (w416:dbl[][])
                    n272 = Array Size(array=w416) -> (size(s)=w415:i32[])
                    n273 = local read "lane num"() -> (w407:i32)
                    n274 = Index Array(array=w415, index=0) -> (element=w413:i32)
                    n275 = Subtract(x=w408, y=w407) -> (x-y=w411:i32)
                    n276 = Decrement(x=w413) -> (x-1=w412:i32)
                    n277 = Subtract(x=w412, y=w411) -> (x-y=w410:i32)
                    n278 = Delete From Array(array=w416, length=w411, index (row)=w410) -> (array with subset deleted=w409:dbl[][])  [unwired: 1 in, 1 out]
                    n279 = local write "lanes"(w409) -> ()
                  }
                }
              }
              frame #2 {
                n280 = local read "lane num"() -> (w419:i32)
                n281 = Less Or Equal?(x=w418, y=w419) -> (x <= y?=w417:bool)
                n282 = case shown="True" w417 {
                  tunnel: w420 -> [w427 _]
                  tunnel: w418 -> [w421 w453]
                  frame True {
                    n283 = Not Equal To 0?(x=w427) -> (x != 0?=w426:bool)
                    n284 = Equal To 0?(x=w421) -> (x = 0?=w425:bool)
                    n285 = Not Equal To 0?(x=w421) -> (x != 0?=w423:bool)
                    n286 = And(x=w426, y=w425) -> (x .and. y?=w422:bool)
                    n287 = Or(x=w423, y=w422) -> (x .or. y?=w424:bool)
                    n288 = case shown="True" w424 {
                      tunnel: w421 -> [_ w432]
                      frame False {
                      }
                      frame True {
                        n289 = local read "lanes"() -> (w438:dbl[][])
                        n290 = local read "lane num"() -> (w428:i32)
                        n291 = Index Array(array=w438, index (row)=0) -> (element=w434:dbl[])  [unwired: 1 in]
                        n292 = Subtract(x=w428, y=w432) -> (x-y=w433:i32)
                        n293 = Index Array(array=w434, index=3) -> (element=w436:dbl)
                        n294 = for {
                          N: w433 -> [_]
                          tunnel: w434 -> [w451]
                          tunnel: w436 -> [w445]
                          shift-right: [w441] -> w429
                          shift-left: dbl[][] [] ("lanes") -> [w440]
                          i -> [w450]
                          n295 = local read "lane width"() -> (w448:dbl)
                          n296 = Increment(x=w450) -> (x+1=w449:i32)
                          n297 = To Double Precision Float(number=w449) -> (double precision float=w447:dbl)
                          n298 = Multiply(x=w448, y=w447) -> (x*y=w446:dbl)
                          n299 = Add(x=w445, y=w446) -> (x+y=w444:dbl)
                          n300 = Replace Array Subset(array=w451, new element #1=w444, index #1=3 ("index"), new element #2=0.0 ("new element/subarray")) -> (w442:dbl[])  [unwired: 1 in]
                          n301 = Build Array (concatenate)(w442, w440) -> (w441:dbl[][])
                        }
                        n302 = Build Array (concatenate)(w429, w438) -> (w437:dbl[][])
                        n303 = local write "lanes"(w437) -> ()
                      }
                    }
                  }
                  frame False {
                    n304 = local read "lane num"() -> (w452:i32)
                    n305 = Subtract(x=w453, y=w452) -> (x-y=w455:i32)
                    n306 = local read "lanes"() -> (w457:dbl[][])
                    n307 = Delete From Array(array=w457, length=w455, index (row)=0) -> (array with subset deleted=w454:dbl[][])  [unwired: 1 in, 1 out]
                    n308 = local write "lanes"(w454) -> ()
                  }
                }
              }
              frame #3 {
                n309 = local read "lanes"() -> (w463:dbl[][])
                n310 = Array Size(array=w463) -> (size(s)=w462:i32[])
                n311 = Index Array(array=w462, index=0) -> (element=w459:i32)
                n312 = Greater?(x=w459, y=1) -> (0:w458:bool)
                n313 = case shown="True" w458 {
                  tunnel: w463 -> [_ w491]
                  frame False {
                    n314 = flat-sequence {
                      frame #0 {
                        w465 = 3.5 ("lane width")
                        n315 = local read "lane num"() -> (w464:i32)
                        n316 = local write "lane width"(w465) -> ()
                        n317 = Multiply(x=0.5, y=w465) -> (x*y=w469:dbl)
                        n318 = for {
                          N: w464 -> [_]
                          tunnel: w465 -> [w490]
                          tunnel: w469 -> [w486]
                          tunnel: [w485] -> w472 mode=indexing
                          i -> [w489]
                          n319 = To Double Precision Float(number=w489) -> (double precision float=w488:dbl)
                          n320 = Multiply(x=w490, y=w488) -> (x*y=w487:dbl)
                          n321 = Add(x=w486, y=w487) -> (x+y=w485:dbl)
                        }
                        n322 = Reverse 1D Array(array=w472) -> (reversed array=w470:dbl[])
                        n323 = Negate(x=w470) -> (-x=w471:dbl[])
                        n324 = Build Array (concatenate)(w471, w472) -> (w473:dbl[])
                        n325 = flat-sequence {
                          tunnel: [w476] -> w466
                          tunnel: w473 -> [w474]
                          tunnel: [w474] -> w467
                          frame #0 {
                            n326 = Divide(x=45.0, y=180.0) -> (x/y=w481:dbl)
                            n327 = Multiply(x=3.141592653589793, y=w481) -> (x*y=w480:dbl)
                            n328 = Absolute Value(x=w474) -> (abs(x)=w475:dbl[])
                            n329 = Tangent(1:w480) -> (0:w479:dbl)
                            n330 = Multiply(x=w475, y=w479) -> (x*y=w478:dbl[])
                            n331 = Add(x=w478, y=3.43) -> (x+y=w476:dbl[])
                          }
                        }
                        n332 = local write "seed_x"(w467) -> ()
                        n333 = local write "seed_y"(w466) -> ()
                      }
                    }
                  }
                  frame True {
                    n334 = Index Array(array=w491, index (col)=3 ("disabled index (col)")) -> (element=w496:dbl[])  [unwired: 1 in]
                    n335 = Negate(x=w496) -> (-x=w497:dbl[])
                    n336 = flat-sequence {
                      tunnel: [w511] -> w493
                      tunnel: w497 -> [w510]
                      frame #0 {
                        n337 = Divide(x=45.0, y=180.0) -> (x/y=w516:dbl)
                        n338 = Multiply(x=3.141592653589793, y=w516) -> (x*y=w515:dbl)
                        n339 = Absolute Value(x=w510) -> (abs(x)=w509:dbl[])
                        n340 = Tangent(1:w515) -> (0:w514:dbl)
                        n341 = Multiply(x=w509, y=w514) -> (x*y=w513:dbl[])
                        n342 = Add(x=w513, y=3.43) -> (x+y=w511:dbl[])
                      }
                    }
                    n343 = for {
                      tunnel: w493 -> [w499] mode=indexing
                      tunnel: w491 -> [w503] mode=indexing
                      tunnel: [w504] -> w495 mode=indexing
                      tunnel: [w499] -> w492 mode=indexing
                      n344 = Multiply(x=w499, y=w499) -> (x*y=w500:dbl)
                      n345 = Multiply(x=w499, y=w500) -> (x*y=w508:dbl)
                      n346 = Array Subset(array=w503, length=4) -> (w501:dbl[])  [unwired: 1 in]
                      n347 = Build Array(w508, w500, w499, 1.0 ("element")) -> (w506:dbl[])
                      n348 = Multiply(x=w501, y=w506) -> (x*y=w505:dbl[])
                      n349 = Add Array Elements(numeric array=w505) -> (sum=w504:dbl)
                    }
                    n350 = local write "seed_y"(w492) -> ()
                    n351 = Negate(x=w495) -> (-x=w494:dbl[])
                    n352 = local write "seed_x"(w494) -> ()
                  }
                }
              }
            }
          }
        }
        frame #7 {
          n353 = disable-structure shown="Disabled" {
            frame Disabled {
              n354 = local read "lanes"() -> (w548:dbl[][])
              n355 = feedback #1(w548) -> (w549:dbl[][])
              n356 = for {
                tunnel: w549 -> [w602] mode=indexing
                tunnel: [w598] -> w527 mode=indexing
                shift-right: [w587] -> w547
                shift-left: w548 -> [w590]
                n357 = Index Array(array=w590, index (col)=3 ("index")) -> (element=w605:dbl[])  [unwired: 1 in]
                n358 = Index Array(array=w602, index=3) -> (element=w606:dbl)
                n359 = Subtract(x=w606, y=w605) -> (x-y=w604:dbl[])
                n360 = local read "lane width"() -> (w596:dbl)
                n361 = Absolute Value(x=w604) -> (abs(x)=w603:dbl[])
                n362 = Array Max & Min(array=w603) -> (min value=w597:dbl, min index (indices)=w589:i32)  [unwired: 2 out]
                n363 = Multiply(x=0.25, y=w596) -> (x*y=w594:dbl)
                n364 = Greater?(x=w594, y=w597) -> (0:w586:bool)
                n365 = case shown="False" w586 {
                  tunnel: w590 -> [w610 w614]
                  tunnel: w589 -> [_ w613]
                  tunnel: [dbl[] [0.0, 0.0, 0.0, 0.0, 0.0] w612] -> w588
                  tunnel: [w610 w611] -> w587
                  frame False {
                  }
                  frame True {
                    n366 = Delete From Array(array=w614, index (row)=w613) -> (deleted portion=w612:dbl[], array with subset deleted=w611:dbl[][])  [unwired: 2 in]
                  }
                }
                n367 = Select(t="Numeric", s=w586, f=1.0) -> (s? t:f=w592:dbl)
                n368 = Decrement(x=w592) -> (x-1=w601:dbl)
                n369 = Multiply(x=w601, y=w588) -> (x*y=w600:dbl[])
                n370 = Multiply(x=w602, y=w592) -> (x*y=w599:dbl[])
                n371 = Subtract(x=w599, y=w600) -> (x-y=w598:dbl[])
              }
              n372 = flat-sequence {
                tunnel: w547 -> [w557]
                tunnel: [w556] -> w546
                frame #0 {
                  n373 = Index Array(array=w557, index (col)=4 ("disabled index (col)")) -> (element=w561:dbl[])  [unwired: 1 in]
                  n374 = Equal?(x=w561, y=1.0) -> (x = y?=w559:bool[])
                  n375 = for {
                    tunnel: w559 -> [w566] mode=indexing
                    shift-right: [w564] -> w556
                    shift-left: dbl[][] [] ("lanes") -> [w565]
                    tunnel: w557 -> [w563] mode=indexing
                    n376 = case shown="False" w566 {
                      tunnel: w565 -> [w567 w570]
                      tunnel: [w567 w569] -> w564
                      tunnel: w563 -> [_ w568]
                      frame False {
                      }
                      frame True {
                        n377 = Build Array (concatenate)(w570, w568) -> (w569:dbl[][])
                      }
                    }
                  }
                }
              }
              n378 = flat-sequence {
                tunnel: w527 -> [w572]
                tunnel: [w571] -> w545
                frame #0 {
                  n379 = Index Array(array=w572, index (col)=4 ("disabled index (col)")) -> (element=w576:dbl[])  [unwired: 1 in]
                  n380 = Greater?(x=w576, y=0.5) -> (0:w574:bool[])
                  n381 = for {
                    tunnel: w574 -> [w581] mode=indexing
                    shift-right: [w579] -> w571
                    shift-left: dbl[][] [] ("lanes") -> [w580]
                    tunnel: w572 -> [w578] mode=indexing
                    n382 = case shown="False" w581 {
                      tunnel: w580 -> [w582 w585]
                      tunnel: [w582 w584] -> w579
                      tunnel: w578 -> [_ w583]
                      frame False {
                      }
                      frame True {
                        n383 = Build Array (concatenate)(w585, w583) -> (w584:dbl[][])
                      }
                    }
                  }
                }
              }
              n384 = Build Array (concatenate)(w546, w545) -> (w544:dbl[][])
              n385 = Index Array(array=w544, index (col) #1=3 ("disabled index (col)"), index (col) #2=0 ("index (col)")) -> (element #1=w542:dbl[], element #2=w540:dbl[], element #3=w539:dbl[], element #4=w538:dbl[], element #5=w537:dbl[], element #6=w536:dbl[])  [unwired: 10 in]
              n386 = Build Cluster Array(w542, w540, w539, w538, w537, w536) -> (w535:cluster{dbl, dbl, dbl, dbl, dbl, dbl}[])
              n387 = Sort 1D Array(array=w535) -> (sorted array=w534:cluster{dbl, dbl, dbl, dbl, dbl, dbl}[])
              n388 = for {
                tunnel: w534 -> [w555] mode=indexing
                tunnel: [w554] -> w533 mode=indexing
                tunnel: [w553] -> w532 mode=indexing
                tunnel: [w552] -> w531 mode=indexing
                tunnel: [w551] -> w530 mode=indexing
                tunnel: [w550] -> w529 mode=indexing
                n389 = Unbundle(w555) -> (w554:dbl, w553:dbl, w552:dbl, w551:dbl, w550:dbl)  [unwired: 1 out]
              }
              n390 = Build Array(w533, w532, w531, w530, w529) -> (w528:dbl[][])
              n391 = Transpose 2D Array(2D array=w528) -> (transposed array=w523:dbl[][])
              n392 = local write "lanes"(w523) -> ()
              n393 = Index Array(array=w523, index (col)=4 ("disabled index (col)")) -> (element=w525:dbl[])  [unwired: 1 in]
              n394 = Multiply(x=w525, y=0.99) -> (x*y=w522:dbl[])
              n395 = Replace Array Subset(array=w523, new element=w522, index (col)=4 ("disabled index (col)")) -> (w520:dbl[][])  [unwired: 1 in]
              n396 = feedback-in #1(w520) -> ()
            }
            frame Enabled {
            }
          }
        }
      }
    }
    frame #2 {
      n397 = Tick Count (ms)() -> (millisecond timer value=w617:u32)
      n398 = Subtract(x=w617, y=w616) -> (x-y=→"time":u32)
    }
    frame #3 {
      n399 = flat-sequence {
        tunnel: [w642] -> w624
        tunnel: [w644] -> w623
        tunnel: w624 -> [w643]
        frame #0 {
          n400 = local read "lanes"() -> (w642:dbl[][])
        }
        frame #1 {
          n401 = for {
            tunnel: [w647] -> w644 mode=indexing
            tunnel: w643 -> [w645] mode=indexing
            n402 = local read "lane_x"() -> (w656:dbl[])
            n403 = Multiply(x=w656, y=w656) -> (x*y=w655:dbl[])
            n404 = Multiply(x=w656, y=w655) -> (x*y=w654:dbl[])
            n405 = Index Array(array=w645, index #1=0 ("index")) -> (element #1=w653:dbl, element #2=w652:dbl, element #3=w651:dbl, element #4=w646:dbl)  [unwired: 3 in]
            n406 = Multiply(x=w654, y=w653) -> (x*y=w650:dbl[])
            n407 = Multiply(x=w655, y=w652) -> (x*y=w649:dbl[])
            n408 = Multiply(x=w656, y=w651) -> (x*y=w648:dbl[])
            n409 = Compound Arithmetic op=ADD(w650, w649, w648, w646) -> (w647:dbl[])
          }
        }
      }
      n410 = local read "lanes"() -> (w621:dbl[][])
      n411 = local read "sensors"() -> (w618:dbl[][])
      n412 = for {
        tunnel: w621 -> [_] mode=indexing
        tunnel: [w641] -> w620 mode=indexing
        n413 = local read "lane_x"() -> (w641:dbl[])
      }
      n414 = local read "sensors"() -> (w619:dbl[][])
      n415 = local read "seed_x"() -> (w639:dbl[])
      n416 = Index Array(array=w618, index (col)=0 ("disabled index (col)")) -> (element=w637:dbl[])  [unwired: 1 in]
      n417 = local read "seed_y"() -> (w632:dbl[])
      n418 = Negate(x=w637) -> (-x=w638:dbl[])
      n419 = Negate(x=w639) -> (-x=w640:dbl[])
      n420 = Index Array(array=w619, index (col)=1 ("disabled index (col)")) -> (element=w628:dbl[])  [unwired: 1 in]
      n421 = call "Convert to Dynamic Data2"("Array"=w628) -> ("Dynamic Data Type"=w629:dynamicdata)  [unwired: 3 in]
      n422 = call "Convert to Dynamic Data4"("Array"=w632) -> ("Dynamic Data Type"=w633:dynamicdata)  [unwired: 3 in]
      n423 = call "Convert to Dynamic Data5"("2D Array"=w620) -> ("Dynamic Data Type"=w625:dynamicdata)  [unwired: 3 in]
      n424 = call "Convert to Dynamic Data"("Array"=w638) -> ("Dynamic Data Type"=w627:dynamicdata)  [unwired: 3 in]
      n425 = call "Convert to Dynamic Data3"("Array"=w640) -> ("Dynamic Data Type"=w631:dynamicdata)  [unwired: 3 in]
      n426 = call "Convert to Dynamic Data6"("2D Array"=w623) -> ("Dynamic Data Type"=w622:dynamicdata)  [unwired: 3 in]
      n427 = Merge Signals(w629, w633, w625) -> (w635:dynamicdata)
      n428 = Merge Signals(w627, w631, w622) -> (w636:dynamicdata)
      n429 = call "Build XY Graph"("Y Input"=w636, "X Input"=w635) -> ("XY Graph"=→"XY Graph":cluster{"Y":dbl[], "Y":dbl[]}[])  [unwired: 3 in, 6 out]
    }
  }
